vi "MTS_Main.vi"() -> ()   [LabVIEW 2010]
panel:
  out "Grid Points":dbl[][](array[numeric])
  in  "Z-Position":dbl=69.999 caption="Z" min=0.0 max=200.0 format="%1.3f um"
  in  "Y-Position":dbl=19.9997 caption="Y" min=0.0 max=200.0 format="%1.3f um"
  in  "X-Position":dbl=48.0021 caption="X" min=0.0 max=200.0 format="%1.3f um"
  in  "Move Stage":bool
  out "Detector4":bool=TRUE
  in  "Measurement Tab Control":T1(tab)
  in  "Measurement Time (s)":i32=60 min=10
  in  "Point Measurement":bool
  in  "Line Time (s)":i32=60 caption="Measurement Time (s)" min=10
  in  "Line Width":dbl=50.0 min=0.1 max=200.0 format="%1.1f um"
  in  "Line Points":u16=100
  in  "Line Scan Axis":enum32{"x-Axis", "y-Axis", "z-Axis"}(ring) caption="Axis"
  in  "Line Scan":bool
  in  "Line Scanner Divider":i32=1 caption="Scanner Divider" min=1 max=10
  in  "Grid Measurement":bool
  in  "Grid Time (s)":i32=2 caption="Time per Point (s)" min=1 max=3600
  in  "Repetitions":u16=1 min=1 max=100
  in  "Z-Axis Offset":dbl=2.0 min=0.1 max=10.0
  in  "Y-Axis Offset":dbl=2.0 min=0.1 max=10.0
  in  "X-Axis Offset":dbl=2.0 min=0.1 max=10.0
  in  "Z-Axis Points":u16=1 min=1 max=100
  in  "Y-Axis Points":u16=50 min=1 max=100
  in  "X-Axis Points":u16=50 min=1 max=100
  out "Grid Time":dbl=91.66666666666667 caption="Measurement Time (min)" format="%#_2f"
  out "Current Grid Point":i32
  in  "Axis":enum32{"x-y", "x-z", "y-z"}(ring)
  in  "Picture size 2":dbl=50.0 min=0.1 max=200.0 format="%1.1f um"
  in  "Picture size":dbl=50.0 min=0.1 max=200.0 format="%1.1f um"
  in  "Axis 2 Pixel":u16=100
  in  "Axis 1 Pixel":u16=100
  in  "Scanner Divider":i32=1 min=1 max=10
  out "Measure. time [s]":i32
  in  "Aquire Image":bool
  out "y":dbl=500.0 format="%.1f nm"
  out "x":dbl=500.0 format="%.1f nm"
  out "Detector3":bool=TRUE
  out "Counts":u32[](array[numeric])
  out "Last Image File No":i32=-1
  out "NxtAutMesPoint":i32
  out "Auto Measure Points":i32
  out "Pattern":dbl[][](array[numeric])
  out "Active pt3":path
  in  "Save Files":bool=TRUE
  out "Intensity (a.u.)":dbl=17475.78930323986 format="%.02f"
  out "Detector2":bool=TRUE
  out "Detector1":bool=TRUE
  out "Excitation":bool=TRUE
  in  "Open MSW":bool
  in  "New MSW":bool
  out "Workspace":path=path "X:/MTusers/Christoph/2011-02-01 Andi/2011-02-01.msw"
  in  "WS File Tree":string(tree)
  out "Stop Measurement":bool
  in  "Learning loop":bool=TRUE
  in  "ShowTab":T2(tab)=enum."TCSPC Histogram"
  out "Video":u8[][](graph)
  in  "Find Mols":bool
  out "Image":i32[][](graph)
  in  "Save Color Image":bool
  in  "psf width [um]":dbl=0.7
  in  "Auto Shutter Control":bool=TRUE
  out "Auto Meas Progress":i32(slide) caption="Point 8 / 15" scale=0.0..15.0
  out "AM image":T3(plugin-control)
  in  "Auto Meas":bool
  in  "Auto Measurement Time (ms)":i32=60 caption="Measurement Time (s)" min=10
  in  "Autopoint-Auto Z":bool
  out "Histogram":i32[][](graph)
  in  "CFD Settings":T4={"Sync Level"=150, "Sync ZeroX"=10, "Sync Offset"=-9000, "Chan Settings"=[{"CHx Level"=50, "CHx ZeroX"=10, "CHx Offset"=400}, {"CHx Level"=50, "CHx ZeroX"=10, "CHx Offset"=400}, {"CHx Level"=150, "CHx ZeroX"=10, "CHx Offset"=19250}, {"CHx Level"=150, "CHx ZeroX"=10, "CHx Offset"=19200}]}
  out "Trace":i32[][](graph)=[[2, 0, 0, 1, 1, 1, 0, 0, 0, 1, 0, 1, 0, 1, 2, 2, 0, 3, 0, 2, 2, 1, 3, 1, 0, 1, 1, 1, 0, 1, 3, 1, 0, 2, 0, 1, 0, 1, 1, 0, 1, 1, 3, 1, 0, 2, 0, 1, 1, 0, 0, 2, 0, 0, 1, 1, 1, 0, 0, 1, 0, 1, 0, 0, 0, 1, 2, 1, 1, 2, 0, 2, 4, 3, 1, 1, 0, 0, 1, 1, 2, 0, 1, 1, 0, 0, 0, 1, 1, 1, 1, 3, 0, 0, 1, 0, 0, 0, 2, 1, 1, 1, 2, 1, 0, 1, 1, 0, 0, 2, 1, 1, 0, 0, 1, 1, 1, 1, 0, 2, 2, 0, 1, 2, 1, 0, 3, 0, 2, 1, 3, 0, 1, 1, 0, 0, 3, 0, 0, 0, 0, 0, 0, 0, 0, 0, 0, 0, 0, 0, 0, 0, 0, 0, 0, 0, 0, 0, 0, 0, 0, 0, 0, 0, 0, 0, 0, 0, 0, 0, 0, 0, 0, 0, 0, 0, 0, 0, 0, 0, 0, 0, 0, 0, 0, 0, 0, 0, 0, 0, 0, 0, 0, 0, 0, 0, 0, 0, 0, 0], [1, 2, 2, 0, 0, 0, 1, 2, 1, 2, 1, 1, 1, 0, 0, 0, 3, 1, 0, 1, 0, 2, 0, 2, 1, 1, 0, 0, 1, 0, 1, 2, 1, 0, 0, 0, 0, 0, 1, 0, 1, 0, 2, 0, 1, 0, 0, 0, 0, 1, 1, 3, 0, 0, 0, 2, 0, 0, 2, 0, 1, 1, 0, 0, 2, 0, 2, 1, 0, 1, 1, 0, 1, 1, 0, 0, 0, 1, 0, 0, 1, 0, 0, 0, 0, 1, 0, 1, 1, 1, 1, 0, 0, 0, 1, 1, 1, 0, 1, 0, 0, 0, 1, 1, 1, 0, 0, 1, 1, 3, 1, 0, 0, 0, 0, 0, 0, 0, 1, 2, 1, 0, 0, 0, 2, 3, 3, 2, 0, 1, 1, 1, 0, 0, 4, 0, 1, 2, 0, 0, 0, 2, 0, 0, 0, 0, 0, 0, 0, 0, 0, 0, 0, 0, 0, 0, 0, 0, 0, 0, 0, 0, 0, 0, 0, 0, 0, 0, 0, 0, 0, 0, 0, 0, 0, 0, 0, 0, 0, 0, 0, 0, 0, 0, 0, 0, 0, 0, 0, 0, 0, 0, 0, 0, 0, 0, 0, 0, 0, 0], [2, 2, 0, 1, 2, 0, 1, 0, 2, 3, 1, 0, 1, 0, 1, 0, 0, 0, 0, 2, 1, 0, 0, 2, 2, 0, 0, 0, 3, 0, 0, 2, 2, 2, 0, 3, 0, 3, 1, 3, 1, 3, 1, 0, 3, 1, 3, 3, 1, 1, 1, 1, 2, 0, 1, 0, 1, 1, 1, 3, 0, 2, 3, 1, 1, 1, 0, 1, 0, 1, 2, 3, 1, 2, 1, 3, 0, 2, 0, 2, 0, 1, 0, 2, 2, 1, 1, 3, 1, 2, 1, 1, 1, 3, 0, 0, 0, 0, 1, 1, 1, 0, 1, 0, 2, 1, 1, 0, 1, 0, 1, 2, 2, 2, 2, 0, 1, 0, 0, 0, 1, 1, 2, 0, 0, 1, 5, 2, 2, 0, 2, 0, 2, 2, 2, 0, 1, 0, 6, 0, 0, 0, 0, 0, 0, 0, 0, 0, 0, 0, 0, 0, 0, 0, 0, 0, 0, 0, 0, 0, 0, 0, 0, 0, 0, 0, 0, 0, 0, 0, 0, 0, 0, 0, 0, 0, 0, 0, 0, 0, 0, 0, 0, 0, 0, 0, 0, 0, 0, 0, 0, 0, 0, 0, 0, 0, 0, 0, 0, 0], [0, 0, 1, 0, 1, 1, 0, 0, 0, 1, 1, 0, 1, 0, 0, 0, 0, 0, 2, 0, 0, 0, 0, 2, 0, 0, 0, 1, 1, 2, 1, 1, 1, 2, 1, 0, 0, 3, 0, 1, 1, 0, 0, 0, 0, 1, 0, 0, 2, 1, 0, 0, 1, 1, 1, 2, 2, 0, 1, 0, 0, 1, 0, 1, 1, 0, 0, 2, 1, 1, 2, 1, 1, 0, 0, 0, 0, 2, 1, 0, 0, 0, 0, 1, 0, 1, 0, 0, 0, 0, 1, 0, 0, 0, 0, 1, 0, 1, 1, 1, 0, 2, 3, 1, 1, 0, 1, 1, 1, 0, 1, 0, 0, 1, 1, 0, 2, 0, 0, 0, 0, 3, 0, 0, 0, 0, 0, 0, 0, 0, 1, 0, 2, 0, 0, 0, 1, 2, 2, 0, 1, 0, 0, 0, 0, 0, 0, 0, 0, 0, 0, 0, 0, 0, 0, 0, 0, 0, 0, 0, 0, 0, 0, 0, 0, 0, 0, 0, 0, 0, 0, 0, 0, 0, 0, 0, 0, 0, 0, 0, 0, 0, 0, 0, 0, 0, 0, 0, 0, 0, 0, 0, 0, 0, 0, 0, 0, 0, 0, 0]]
  out "FiFo Overrun":bool
  in  "SCANNER EMERGENCY":bool
  out "Do Measurement":T5(ring)
  in  "Settings":bool
  in  "PI E710 Port":u16(ring) items=["COM1", "COM2", "COM3", "COM4", "COM5", "COM6", "COM7", "COM8", "COM9"]
  out "MeasRunig":bool
  in  "Stop Program":bool
  out "Global Stop":bool=TRUE
  # "Workspace"
  # "Shutter:"
  # "Point Measurement Settings"
  # "Point Position"
  # "Line Scan Settings"
  # "Starting Point"
  # "Grid Measurement Settings"
  # "Starting Point"
  # "um"
  # "um"
  # "um"
  # "Image Scan Settings"
  # "Upper Left"
  # "Pixelsize"
  # "Auto Measurement Settings"
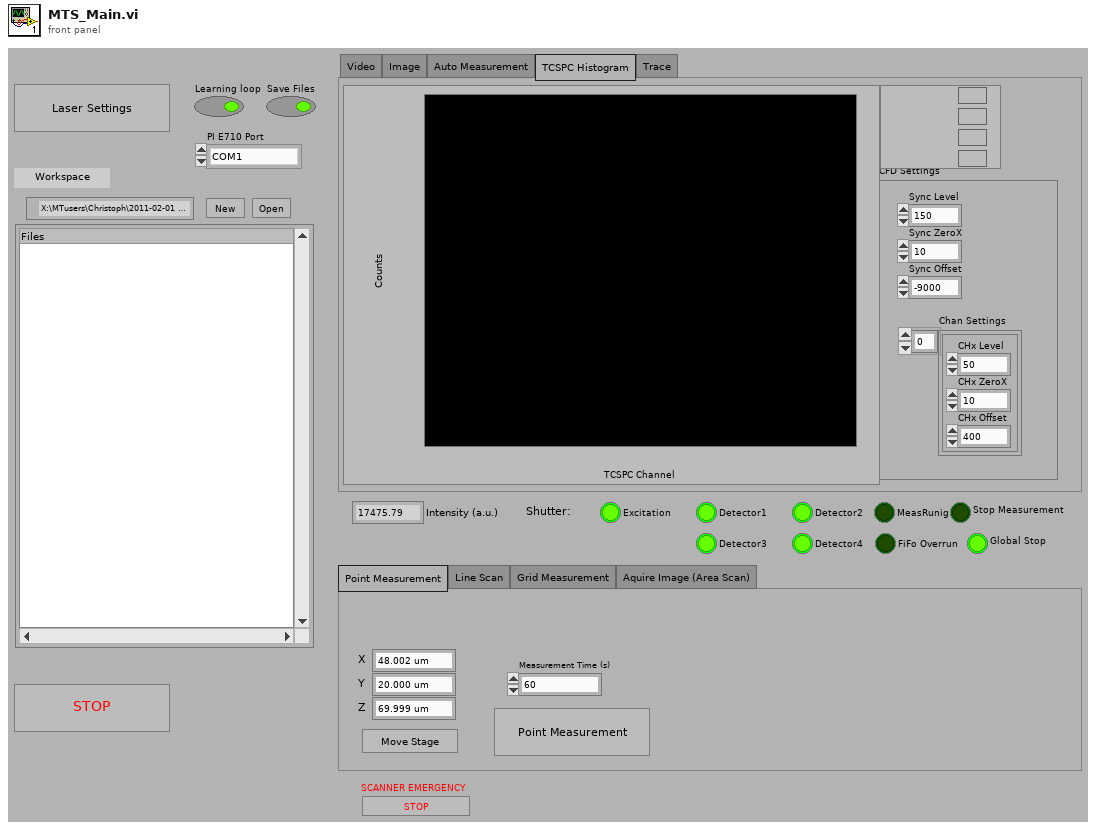
[diagram p1: front panel]
types:
  T1 = enum32{"Point Measurement", "Line Scan", "Grid Measurement", "Aquire Image (Area Scan)"}
  T2 = enum32{"Video", "Image", "Auto Measurement", "TCSPC Histogram", "Trace"}
  T3 = typedef "IMAQ Image.ctl" = refnum<image>
  T4 = cluster{"Sync Level":i32, "Sync ZeroX":i32, "Sync Offset":i32, "Chan Settings":cluster{"CHx Level":i32, "CHx ZeroX":i32, "CHx Offset":i32}[]}
  T5 = enum16{"No Measurement", "Aquire Image", "Point Measurement", "Multi Measurement", "Save Color Image", "Find Single Mol.", "Auto Measurement Control", "Auto Point", "Aquire Line Scan", "Grid Measurement"}
  T6 = cluster{"Position":cluster{"X-Position":dbl, "Y-Position":dbl, "Z-Position":dbl}, "Picture Size Axis 1":dbl, "Picture Size Axis 2":dbl, "Axis":i32, "Axis 1 Pixels":u16, "Axis 2 Pixels":u16, "Scanner Divider":i32}
  T7 = enum16{"CAN_Baud_1M", "CAN_BAUD_500K", "CAN_BAUD_250K", "CAN_BAUD_125K", "CAN_BAUD_100K", "CAN_BAUD_50K", "CAN_BAUD_20K", "CAN_BAUD_10K", "CAN_BAUD_5K", "User"}
  T8 = typedef "Image Type" = u32
  T9 = cluster{"Height":u32, "Width":u32, "Pixel Depth":u32}
  T10 = cluster{"Dev":i32, "SerNo":string, "HW_Model":string, "HW_Partno":string}[]
  T11 = enum32{"Video", "Image", "TCSPC Histogram", "Trace"}
  T12 = cluster{"ID":u32, "MSG type":enum8{"STD, NO RTR", "STD,RTR", "XTD, NO RTR", "XTD, RTR"}, "LEN":u8, "DATA":u8[]}
  T13 = enum32{"Invalid", "Standard", "Closed", "Hidden", "Minimized", "Maximized"}
  T14 = enum16{"No Measurement", "Aquire Image", "Point Measurement", "Multi Measurement", "Save Color Image"}
  T15 = enum16{"No Measurement", "Aquire Image", "Point Measurement", "Multi Measurement", "Save Color Image", "Find Single Mol.", "Auto Measurement Control", "Auto Point", "Aquire Line Scan"}
  T16 = enum16{"No Measurement", "Aquire Image", "Point Measurement", "Multi Measurement", "Save Color Image", "Find Single Mol.", "Auto Measurement Control", "Auto Point"}
  T17 = enum16{"No Measurement", "Aquire Image", "Point Measurement", "Multi Measurement", "Save Color Image", "Find Single Mol."}
  T18 = enum16{"Get (Default)", "Set Workspace", "Append File", "Change Comment"}
  T19 = enum16{"unknown", "pt3 File", "png Image", "bmp Image"}
  T20 = enum32{"Bad", "Idle", "Run top level", "Running"}
  T21 = cluster{"File No":i32, "File Path":path, "Parent File":i32, "File Type":enum16{"unknown", "pt3 File", "png Image", "bmp Image"}, "Measurement Type":enum16{"not a pt3 File", "Image File", "Point Measurement", "Auto Point", "Line Scan", "Grid Scan"}, "Upper Left":cluster{"x-Position":dbl, "y-Position":dbl, "z-Position":dbl}, "Pixels":i32[], "Picture Size":dbl[], "Scan Axis":enum32{"x-y", "x-z", "y-z"}}[]
  T22 = typedef "LVPoint32TypeDef.ctl" = cluster{"Horizontal":i32, "Vertical":i32}
  T23 = cluster{"Shift":bool, "Ctrl":bool, "Alt":bool, "Cmd":bool, "Opt":bool}
  T24 = cluster{"File No":i32, "File Path":path, "Parent File":i32, "File Type":enum16{"unknown", "pt3 File", "png Image", "bmp Image"}, "Measurement Type":enum16{"not a pt3 File", "Image File", "Point Measurement", "Auto Point", "Line Scan", "Grid Scan"}, "Upper Left":cluster{"x-Position":dbl, "y-Position":dbl, "z-Position":dbl}, "Pixels":i32[], "Picture Size":dbl[], "Scan Axis":enum32{"x-y", "x-z", "y-z"}}
  T25 = enum16{"not a pt3 File", "Image File", "Point Measurement", "Auto Point", "Line Scan", "Grid Scan"}
  T26 = cluster{"x-Position":dbl, "y-Position":dbl, "z-Position":dbl}
  T27 = cluster{"Upper Left":cluster{"x-Position":dbl, "y-Position":dbl, "z-Position":dbl}, "value":dbl, "value":dbl, "Scan Axis":enum32{"x-y", "x-z", "y-z"}, "value":i32, "value":i32, "index":i32}
  T28 = cluster{"ID":u32, "MSG type":enum8{"STD, NO RTR", "STD,RTR", "XTD, NO RTR", "XTD, RTR"}, "LEN":u8, "Data":u8[]}
  T29 = enum16{"not a pt3 File", "Image File", "Point Measurement", "Auto Point", "Line Scan"}
  T30 = enum16{"not a pt3 File", "Image File", "Point Measurement", "Auto Point"}
  T31 = cluster{"X-Position":dbl, "Y-Position":dbl, "Z-Position":dbl}
  T32 = cluster{"Dev":i32, "SerNo":string, "HW_Model":string, "HW_Partno":string}
  T33 = cluster{"Comment":string, "Binning":i32, "Offset":i32, "AcquisitionTime (ms)":i32, "HardwareSerial":i32, "SyncDivider":i32, "Resolution (ps)":dbl, "InpRate0":i32, "InpRate1":i32, "CFD Settings":cluster{"Sync Level":i32, "Sync ZeroX":i32, "Sync Offset":i32, "Chan Settings":cluster{"CHx Level":i32, "CHx ZeroX":i32, "CHx Offset":i32}[]}, "ModuleInfo":cluster{"modelcode":i32, "versioncode":i32}[], "BaseResolution (ps)":dbl, "RefClockSource":i32, "ChanInfo":cluster{"CHx Level":i32, "CHx ZeroX":i32, "CHx Offset":i32, "CHx modidx":i32}[], "SyncRate":i32, "InputsEnabled":i64}
  T34 = cluster{"Dimensions":i32, "Time Per Pixel [ms]":dbl, "Acceleration":i32, "Pattern":i32, "X0":sgl, "Y0":sgl, "PixX":i32, "PixY":i32, "PixResol":sgl, "TStartTo":sgl, "TStoptTo":sgl, "TStartFro":sgl, "TStopFro":sgl}
  T35 = cluster{"InpRateFilePos":i64, "StopAfterFilePos":i64}
  T36 = cluster{"Picture Size":dbl[], "Pixels":i32[], "Upper Left":cluster{"x-Position":dbl, "y-Position":dbl, "z-Position":dbl}}
  T37 = cluster{"Ident":string, "Format Version":string, "Creator Name":string, "Creator Version":string, "File Time":string, "Comment":string, "Binning":i32, "Offset":i32, "AcquisitionTime (ms)":i32, "HardwareSerial":i32, "SyncDivider":i32, "Resolution (ps)":dbl, "InpRate0":i32, "InpRate1":i32, "CFD Settings":cluster{"Sync Level":i32, "Sync ZeroX":i32, "Sync Offset":i32, "Chan Settings":cluster{"CHx Level":i32, "CHx ZeroX":i32, "CHx Offset":i32}[]}}
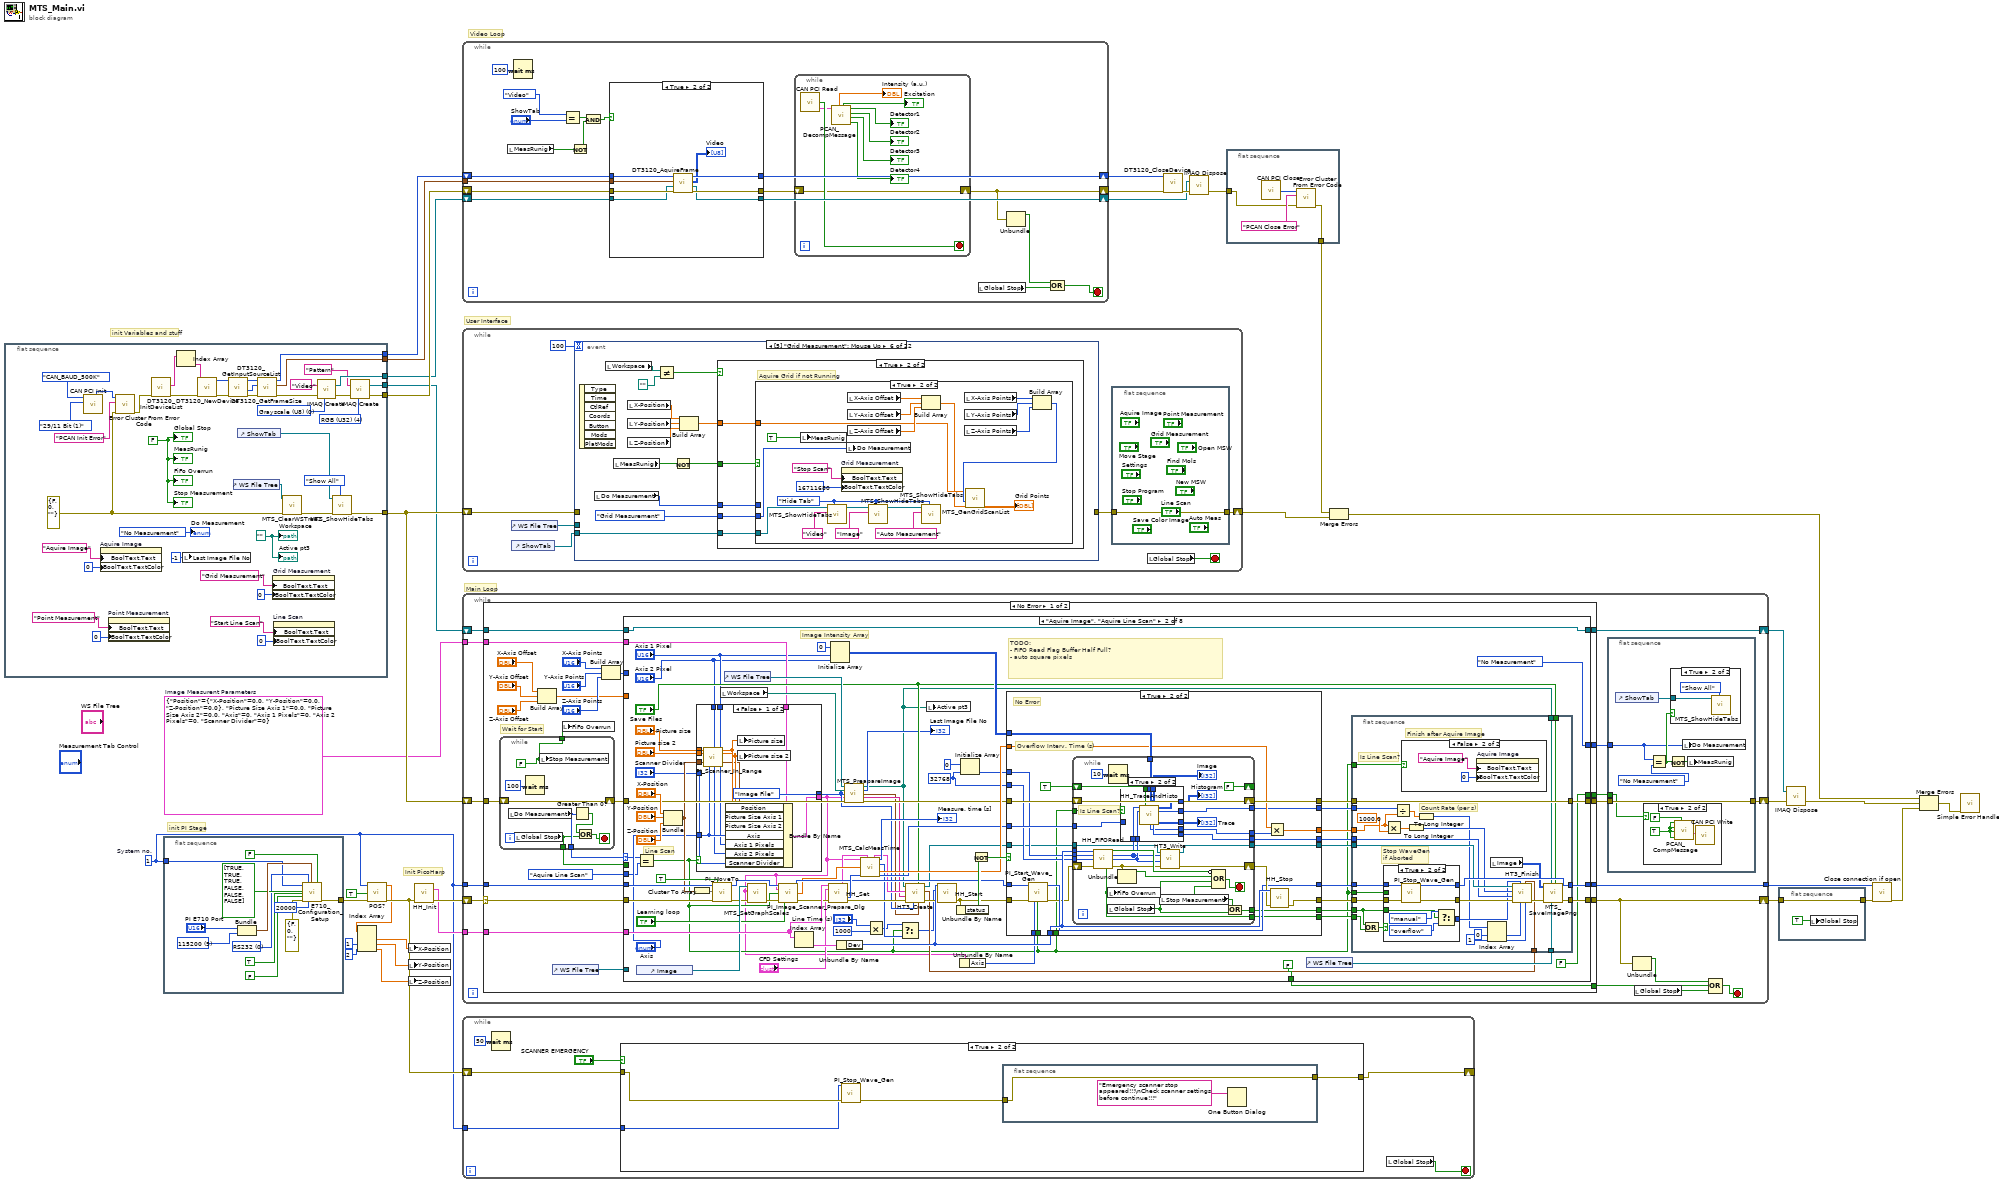
[diagram p0: block diagram]
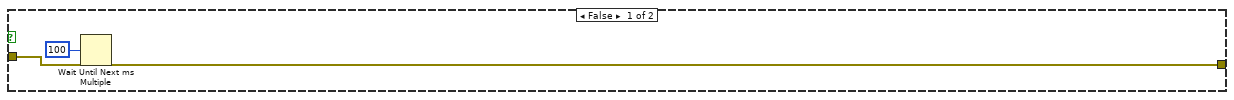
[diagram p3: hidden frame]
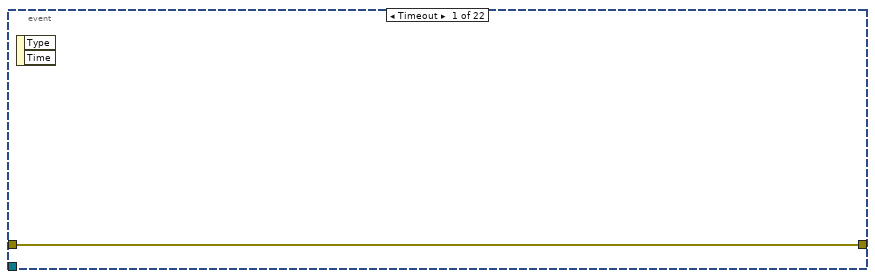
[diagram p4: hidden frame]
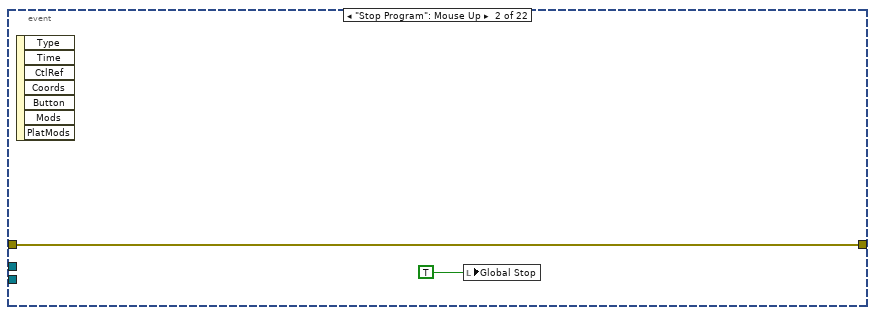
[diagram p5: hidden frame]
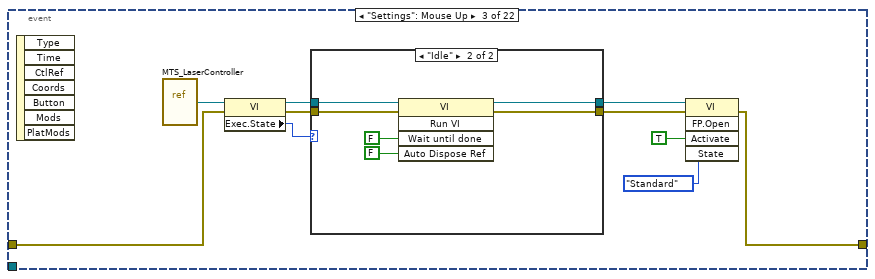
[diagram p6: hidden frame]
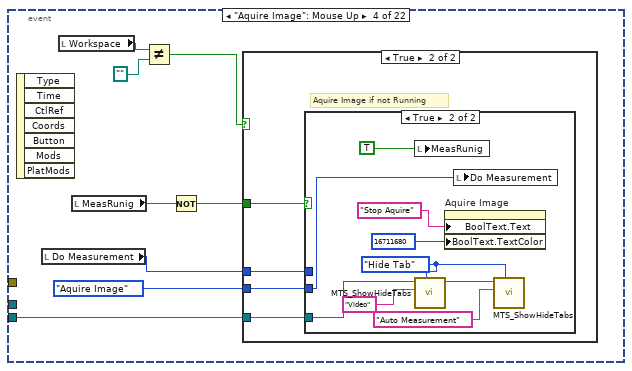
[diagram p8: hidden frame]
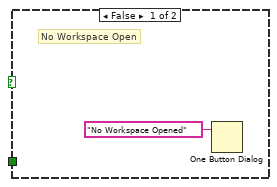
[diagram p9: hidden frame]
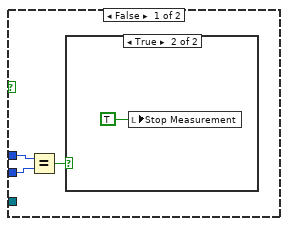
[diagram p10: hidden frame]
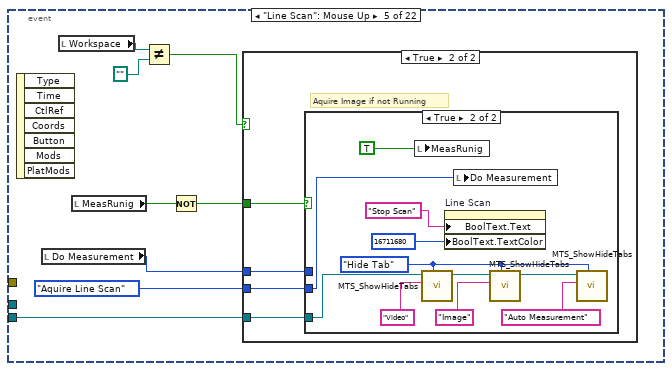
[diagram p12: hidden frame]
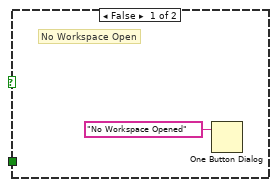
[diagram p13: hidden frame]
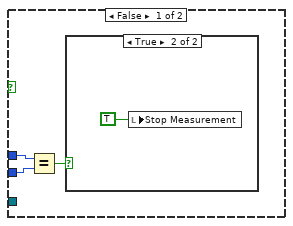
[diagram p14: hidden frame]
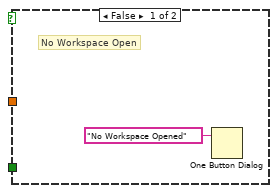
[diagram p16: hidden frame]
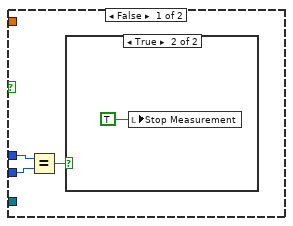
[diagram p17: hidden frame]
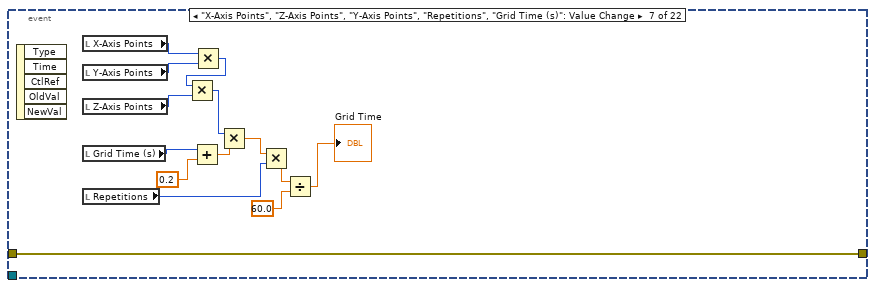
[diagram p19: hidden frame]
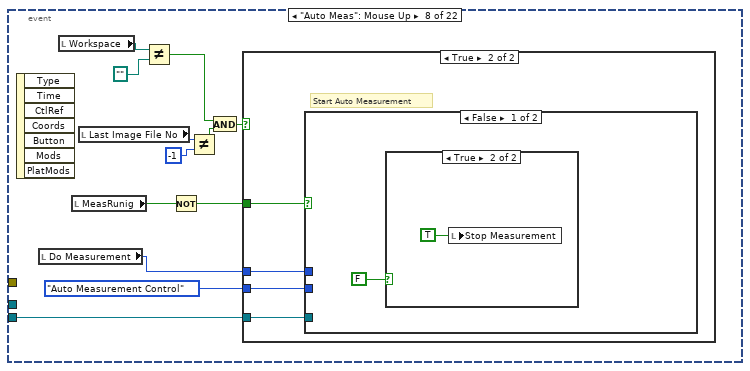
[diagram p20: hidden frame]
diagram:
  w1 = T6 {"Position"={"X-Position"=0.0, "Y-Position"=0.0, "Z-Position"=0.0}, "Picture Size Axis 1"=0.0, "Picture Size Axis 2"=0.0, "Axis"=0, "Axis 1 Pixels"=0, "Axis 2 Pixels"=0, "Scanner Divider"=0}  # Image Measurent Parameters
  w8 = 1  # System no.
  # "Video Loop"
  # "Init PicoHarp"
  # "init Variables and stuff"
  # "User Interface"
  # "init PI Stage"
  # "Main Loop"
  n1 = flat-sequence {
    tunnel: [w61] -> w32
    tunnel: [w51] -> w27
    tunnel: [w68] -> w25
    tunnel: [w65] -> w21
    tunnel: [w50] -> w20
    tunnel: [w47] -> w12
    frame #0 {
      w48 = T8 4 items=["Grayscale (U8)", "Grayscale (I16)", "Grayscale (SGL)", "Complex (CSG)", "RGB (U32)", "HSL (U32)", "RGB (U64)", "Grayscale (U16)"] ("Image Type")
      w66 = T8 0 items=["Grayscale (U8)", "Grayscale (I16)", "Grayscale (SGL)", "Complex (CSG)", "RGB (U32)", "HSL (U32)", "RGB (U64)", "Grayscale (U16)"] ("Image Type")
      w41 = path ""
      w55 = errorcluster {"status"=FALSE, "code"=0, "source"=""} ("error in")
      w77 = FALSE ("Global Stop")
      n2 = call "CAN PCI Init.vi"("CAN Msg Type"=enum16{"11 Bit (0)", "29/11 Bit (1)"}."29/11 Bit (1)", "BTR0BTR1"=T7."CAN_BAUD_500K") -> ("Error Number"=w56:u32)  [unwired: 7 in, 2 out]
      n3 = property on="Aquire Image" class="Bool"("BoolText.Text"="Aquire Image" ("Caption.Text"), "BoolText.TextColor"=u32 0 ("Boolean Text.Colors:FG Color")) -> ()  [unwired: 2 in, 2 out]
      n4 = property on="Point Measurement" class="Bool"("BoolText.Text"="Point Measurement" ("Caption.Text"), "BoolText.TextColor"=u32 0 ("Boolean Text.Colors:FG Color")) -> ()  [unwired: 2 in, 2 out]
      n5 = call <vilib>:"Error Cluster From Error Code.vi"("error in (no error)"=w55, "error message (\"\")"="PCAN Init Error" ("error message (\"\")"), "error code (0)"=w56) -> ("error out"=w54:errorcluster)  [unwired: 6 in]
      n6 = call "DT3120_InitDeviceList.vi"("error in (no error)"=w54) -> ("error out"=w75:errorcluster, "Alias List"=w76:string[])  [unwired: 9 out]
      n7 = Index Array(array=w76) -> (element=w74:string)  [unwired: 1 in]
      n8 = local write "Last Image File No"(-1 ("Last Image File No")) -> ()
      n9 = call "DT3120_NewDevice.vi"("error in (no error)"=w75, "Alias"=w74) -> ("error out"=w70:errorcluster, "DevId"=w69:i32)  [unwired: 8 out]
      n10 = call "DT3120_GetInputSourceList.vi"("error in (no error)"=w70, "DevId"=w69) -> ("error out"=w73:errorcluster, "Active Source"=w72:u16, "DevId (dup)"=w71:i32)  [unwired: 7 out]
      n11 = control-ref of="WS File Tree"() -> (w63:refnum<vi>)
      n12 = control-ref of="ShowTab"() -> (w60:refnum<vi>)
      n13 = call "DT3120_GetFrameSize.vi"("error in (no error)"=w73, "Source"=w72, "DevId"=w71) -> ("error out"=w67:errorcluster, "Frame Size"=w65:T9, "DevId (dup)"=w68:i32)  [unwired: 6 in]
      n14 = property on="Grid Measurement" class="Bool"("BoolText.Text"="Grid Measurement" ("Caption.Text"), "BoolText.TextColor"=u32 0 ("Boolean Text.Colors:FG Color")) -> ()  [unwired: 2 in, 2 out]
      n15 = property on="Line Scan" class="Bool"("BoolText.Text"="Start Line Scan" ("Caption.Text"), "BoolText.TextColor"=u32 0 ("Boolean Text.Colors:FG Color")) -> ()  [unwired: 2 in, 2 out]
      n16 = call "MTS_ClearWSTree2.vi"("error in"=w55, "Tree Refnum"=w63) -> ("error out"=w62:errorcluster)  [unwired: 8 in, 1 out]
      n17 = call "IMAQ Create"("Image Name"="Video", "Image Type"=w66, "error in (no error)"=w67) -> ("New Image"=w50:T3, "error out"=w52:errorcluster)  [unwired: 2 in]
      n18 = call "MTS_ShowHideTabs.vi"("Action"=enum16{"Show All", "Hide Tab", "Show Tab"}."Show All", "error in (no error)"=w62, "ShowTab"=w60) -> ("error out"=w61:errorcluster)  [unwired: 7 in, 1 out]
      n19 = call "IMAQ Create"("Image Name"="Pattern", "Image Type"=w48, "error in (no error)"=w52) -> ("New Image"=w47:T3, "error out"=w51:errorcluster)  [unwired: 2 in]
      "Global Stop" <- w77
      "MeasRunig" <- w77
      "Do Measurement" <- T5."No Measurement" ("Do Measurement")
      "FiFo Overrun" <- w77
      "Stop Measurement" <- w77
      "Workspace" <- w41
      "Active pt3" <- w41
    }
  }
  n20 = flat-sequence {
    tunnel: [w81] -> w11
    tunnel: w8 -> [w80]
    frame #0 {
      w88 = u16 5 items=["9600", "14400", "19200", "38400", "57600", "115200"] ("Baudrate")
      w83 = u16 0 items=["RS232", "GPIB"] ("Interface")
      n21 = Bundle("PI E710 Port"="PI E710 Port", "Baudrate"=w88) -> (w89:cluster{"PI E710 Port":u16, "Baudrate":u16})  [unwired: 1 out]
      n22 = call <userlib>:"E710_Configuration_Setup.vi"("System no."=w80, "Are stages connected?"=bool[] [TRUE, TRUE, TRUE, FALSE, FALSE, FALSE], "Change servo \nstatus to ON?"=TRUE ("Change servo \nstatus to ON?"), "Perform autozero?"=FALSE ("All axes?"), "error in"=errorcluster {"status"=FALSE, "code"=0, "source"=""}, "Interface"=w83, "Timeout"=u32 20000, "RS232 settings"=w89, "Move to middle?"=FALSE) -> ("error out"=w81:errorcluster)  [unwired: 3 in, 7 out]
    }
  }
  n23 = call <userlib>:"POS?.vi"("System no."=w8, "All axes?"=TRUE, "error in"=w11) -> ("Position"=w7:dbl[], "error out"=w10:errorcluster)  [unwired: 2 in, 13 out]
  n24 = Index Array(array=w7, index #2=1 ("index"), index #3=2 ("index")) -> (element #1=w3:dbl, element #2=w2:dbl, element #3=w4:dbl)  [unwired: 1 in]
  n25 = local write "X-Position"(w3) -> ()
  n26 = local write "Y-Position"(w2) -> ()
  n27 = local write "Z-Position"(w4) -> ()
  n28 = call "HH_Init.vi"("error in (no error)"=w10) -> ("Device List"=w30:T10, "error out"=w31:errorcluster)  [unwired: 12 in, 1 out]
  n29 = while {
    shift-right: [w90] -> w26
    shift-left: w27 -> [w104]
    shift-right: [w97] -> w24
    shift-left: w25 -> [w98]
    tunnel: w21 -> [w99]
    shift-right: [w96] -> w18
    shift-left: w20 -> [w100]
    stop <- w103 stop-if-true
    n30 = local read "MeasRunig"() -> (w95:bool)
    n31 = Wait (ms)(milliseconds to wait=u32 100) -> ()  [unwired: 1 out]
    n32 = Equal?(x=T11."Video" ("ShowTab"), y="ShowTab") -> (x = y?=w94:bool)
    n33 = Not(x=w95) -> (.not. x?=w92:bool)
    n34 = And(x=w94, y=w92) -> (x .and. y?=w93:bool)
    n35 = case shown="True" w93 {
      tunnel: w104 -> [w119 w127]
      tunnel: [w119 w126] -> w91
      tunnel: w100 -> [w117 w125]
      tunnel: w99 -> [_ w124]
      tunnel: w98 -> [w118 w123]
      tunnel: [w118 w122] -> w97
      tunnel: [w117 w121] -> w96
      frame False {
      }
      frame True {
        n36 = call "DT3120_AquireFrame.vi"("error in (no error)"=w127, "Image"=w125, "Frame Size"=w124, "DevId"=w123) -> ("error out"=w126:errorcluster, "Image Out"=w121:T3, "Frame"=→"Video":u8[][], "DevId (dup)"=w122:i32)  [unwired: 4 in]
      }
    }
    n37 = while {
      shift-right: [w114] -> w90
      shift-left: w91 -> [w114]
      stop <- w116 stop-if-true
      n38 = call "CAN PCI Read.vi"() -> ("RcvQueueEmpty"=w116:bool, "CAN_Message out"=w115:T12)  [unwired: 1 in, 1 out]
      n39 = call "PCAN_DecompMessage.vi"("CAN_Message out"=w115) -> ("Detector4 Shutter Open?"=→"Detector4":bool, "Detector3 Shutter Open?"=→"Detector3":bool, "Detector2 Shutter Open?"=→"Detector2":bool, "Detector1 Shutter Open?"=→"Detector1":bool, "Excitation Shutter Open?"=→"Excitation":bool, "Intensity (a.u.)"=→"Intensity (a.u.)":dbl)  [unwired: 3 in, 2 out]
    }
    n40 = local read "Global Stop"() -> (w102:bool)
    n41 = Unbundle(w90) -> ("status"=w101:bool)  [unwired: 2 out]
    n42 = Compound Arithmetic op=OR(w101, w102) -> (w103:bool)
  }
  n43 = while {
    shift-right: [w132] -> w23
    shift-left: w32 -> [w133]
    stop <- w130 stop-if-true
    n44 = control-ref of="WS File Tree"() -> (w129:refnum<vi>)
    n45 = control-ref of="ShowTab"() -> (w128:refnum<vi>)
    n46 = event shown="[5] \"Grid Measurement\": Mouse Up" {
      selector: _ -> [_ _ _ _ _ _ _ _ _ _ _ _ _ _ _ _ _ _ _ _ _ _]
      dyn-events: _ -> [_ _ _ _ _ _ _ _ _ _ _ _ _ _ _ _ _ _ _ _ _ _]
      timeout: 100 -> [_ _ _ _ _ _ _ _ _ _ _ _ _ _ _ _ _ _ _ _ _ _]
      tunnel: w133 -> [w136 w138 w147 _ _ _ w267 _ _ _ _ _ w354 w390 _ w442 _ _ _ _ _ _]
      tunnel: [w136 w138 w139 _ _ _ w267 _ _ _ _ _ w352 w387 _ w441 _ _ _ _ _ _] -> w131
      tunnel: w129 -> [_ _ _ _ _ _ _ _ _ _ _ _ w356 w391 _ _ _ _ _ _ _ _]
      tunnel: w128 -> [_ _ _ w157 w184 w216 _ w274 w293 w301 w309 w337 _ _ _ _ _ _ _ _ _ _]
      event Timeout {
        n47 = event-data() -> ()  [unwired: 1 in, 2 out]
      }
      event "Stop Program": Mouse Up {
        n48 = event-data() -> ()  [unwired: 1 in, 7 out]
        n49 = local write "Global Stop"(TRUE ("Global Stop")) -> ()
      }
      event "Settings": Mouse Up {
        n50 = event-data() -> ()  [unwired: 1 in, 7 out]
        n51 = vi-ref "MTS_LaserController.vi"() -> (w148:refnum<vi>)
        n52 = property class="VI"(reference=w148, error in=w147) -> (reference out=w145:refnum<vi>, error out=w146:errorcluster, "Exec.State"=w144:T20)
        n53 = case shown="\"Idle\"" w144 {
          tunnel: w146 -> [w150 w156]
          tunnel: w145 -> [w149 w155]
          tunnel: [w150 w152] -> w143
          tunnel: [w149 w151] -> w142
          frame "Bad", Default {
          }
          frame "Idle" {
            n54 = invoke class="VI" method="Run VI"(reference=w155, error in=w156, "Wait until done"=FALSE ("Wait Until Done"), "Auto Dispose Ref"=FALSE ("Auto Dispose Reference")) -> (reference out=w151:refnum<vi>, error out=w152:errorcluster)  [unwired: 1 in, 3 out]
          }
        }
        n55 = invoke class="VI" method="FP.Open"(reference=w142, error in=w143, "Activate"=TRUE ("Activate?"), "State"=T13."Standard") -> (error out=w139:errorcluster)  [unwired: 1 in, 4 out]
      }
      event "Aquire Image": Mouse Up {
        n56 = event-data() -> ()  [unwired: 1 in, 7 out]
        n57 = local read "Do Measurement"() -> (w161:T5)
        n58 = local read "Workspace"() -> (w160:path)
        n59 = local read "MeasRunig"() -> (w164:bool)
        n60 = Not Equal?(x=w160, y=path "") -> (x != y?=w158:bool)
        n61 = Not(x=w164) -> (.not. x?=w163:bool)
        n62 = case shown="True" w158 {
          tunnel: w163 -> [_ w169]
          tunnel: T14."Aquire Image" ("Do Measurement") -> [_ w168]
          tunnel: w161 -> [_ w167]
          tunnel: w157 -> [_ w166]
          frame False {
            # "No Workspace Open"
            n63 = One Button Dialog(message="No Workspace Opened") -> ()  [unwired: 1 in, 1 out]
          }
          frame True {
            # "Aquire Image if not Running"
            n64 = case shown="True" w169 {
              tunnel: w168 -> [w171 w180]
              tunnel: w167 -> [w172 _]
              tunnel: w166 -> [_ w177]
              frame False {
                n65 = Equal?(x=w172, y=w171) -> (x = y?=w170:bool)
                n66 = case shown="True" w170 {
                  frame False {
                  }
                  frame True {
                    n67 = local write "Stop Measurement"(TRUE ("Stop Measurement")) -> ()
                  }
                }
              }
              frame True {
                w175 = enum16{"Show All", "Hide Tab", "Show Tab"}."Hide Tab" ("Action")
                n68 = local write "MeasRunig"(TRUE ("Measurement Running")) -> ()
                n69 = call "MTS_ShowHideTabs.vi"("Action"=w175, "Tab Caption"="Video", "ShowTab"=w177) -> ("ShowTab (dup)"=w176:refnum<vi>)  [unwired: 7 in, 1 out]
                n70 = property on="Aquire Image" class="Bool"("BoolText.Text"="Stop Aquire" ("Caption.Text"), "BoolText.TextColor"=u32 16711680 ("Boolean Text.Colors:FG Color")) -> ()  [unwired: 2 in, 2 out]
                n71 = local write "Do Measurement"(w180) -> ()
                n72 = call "MTS_ShowHideTabs.vi"("Action"=w175, "Tab Caption"="Auto Measurement", "ShowTab"=w176) -> ()  [unwired: 7 in, 2 out]
              }
            }
          }
        }
      }
      event "Line Scan": Mouse Up {
        n73 = event-data() -> ()  [unwired: 1 in, 7 out]
        n74 = local read "Do Measurement"() -> (w188:T5)
        n75 = local read "Workspace"() -> (w187:path)
        n76 = local read "MeasRunig"() -> (w190:bool)
        n77 = Not Equal?(x=w187, y=path "") -> (x != y?=w185:bool)
        n78 = Not(x=w190) -> (.not. x?=w189:bool)
        n79 = case shown="True" w185 {
          tunnel: w189 -> [_ w195]
          tunnel: T15."Aquire Line Scan" ("Do Measurement") -> [_ w194]
          tunnel: w188 -> [_ w193]
          tunnel: w184 -> [_ w192]
          frame False {
            # "No Workspace Open"
            n80 = One Button Dialog(message="No Workspace Opened") -> ()  [unwired: 1 in, 1 out]
          }
          frame True {
            # "Aquire Image if not Running"
            n81 = case shown="True" w195 {
              tunnel: w194 -> [w197 w208]
              tunnel: w193 -> [w198 _]
              tunnel: w192 -> [_ w205]
              frame False {
                n82 = Equal?(x=w198, y=w197) -> (x = y?=w196:bool)
                n83 = case shown="True" w196 {
                  frame False {
                  }
                  frame True {
                    n84 = local write "Stop Measurement"(TRUE ("Stop Measurement")) -> ()
                  }
                }
              }
              frame True {
                w200 = enum16{"Show All", "Hide Tab", "Show Tab"}."Hide Tab" ("Action")
                n85 = local write "MeasRunig"(TRUE ("Measurement Running")) -> ()
                n86 = call "MTS_ShowHideTabs.vi"("Action"=w200, "Tab Caption"="Video", "ShowTab"=w205) -> ("ShowTab (dup)"=w203:refnum<vi>)  [unwired: 7 in, 1 out]
                n87 = property on="Line Scan" class="Bool"("BoolText.Text"="Stop Scan" ("Caption.Text"), "BoolText.TextColor"=u32 16711680 ("Boolean Text.Colors:FG Color")) -> ()  [unwired: 2 in, 2 out]
                n88 = local write "Do Measurement"(w208) -> ()
                n89 = call "MTS_ShowHideTabs.vi"("Action"=w200, "Tab Caption"="Image", "ShowTab"=w203) -> ("ShowTab (dup)"=w201:refnum<vi>)  [unwired: 7 in, 1 out]
                n90 = call "MTS_ShowHideTabs.vi"("Action"=w200, "Tab Caption"="Auto Measurement", "ShowTab"=w201) -> ()  [unwired: 7 in, 2 out]
              }
            }
          }
        }
      }
      event "Grid Measurement": Mouse Up {
        n91 = event-data() -> ()  [unwired: 1 in, 7 out]
        n92 = local read "Do Measurement"() -> (w220:T5)
        n93 = local read "Workspace"() -> (w219:path)
        n94 = local read "MeasRunig"() -> (w222:bool)
        n95 = local read "X-Position"() -> (w212:dbl)
        n96 = local read "Y-Position"() -> (w213:dbl)
        n97 = local read "Z-Position"() -> (w214:dbl)
        n98 = Not Equal?(x=w219, y=path "") -> (x != y?=w217:bool)
        n99 = Not(x=w222) -> (.not. x?=w221:bool)
        n100 = Build Array(w212, w213, w214) -> (w211:dbl[])
        n101 = case shown="True" w217 {
          tunnel: w221 -> [_ w228]
          tunnel: T5."Grid Measurement" ("Do Measurement") -> [_ w227]
          tunnel: w220 -> [_ w226]
          tunnel: w216 -> [_ w225]
          tunnel: w211 -> [_ w224]
          frame False {
            # "No Workspace Open"
            n102 = One Button Dialog(message="No Workspace Opened") -> ()  [unwired: 1 in, 1 out]
          }
          frame True {
            # "Aquire Grid if not Running"
            n103 = case shown="True" w228 {
              tunnel: w227 -> [w230 w251]
              tunnel: w226 -> [w231 _]
              tunnel: w225 -> [_ w248]
              tunnel: w224 -> [_ w234]
              frame False {
                n104 = Equal?(x=w231, y=w230) -> (x = y?=w229:bool)
                n105 = case shown="True" w229 {
                  frame False {
                  }
                  frame True {
                    n106 = local write "Stop Measurement"(TRUE ("Stop Measurement")) -> ()
                  }
                }
              }
              frame True {
                w243 = enum16{"Show All", "Hide Tab", "Show Tab"}."Hide Tab" ("Action")
                n107 = local write "MeasRunig"(TRUE ("Measurement Running")) -> ()
                n108 = call "MTS_ShowHideTabs.vi"("Action"=w243, "Tab Caption"="Video", "ShowTab"=w248) -> ("ShowTab (dup)"=w246:refnum<vi>)  [unwired: 7 in, 1 out]
                n109 = property on="Grid Measurement" class="Bool"("BoolText.Text"="Stop Scan" ("Caption.Text"), "BoolText.TextColor"=u32 16711680 ("Boolean Text.Colors:FG Color")) -> ()  [unwired: 2 in, 2 out]
                n110 = local write "Do Measurement"(w251) -> ()
                n111 = local read "X-Axis Offset"() -> (w242:dbl)
                n112 = local read "Y-Axis Offset"() -> (w241:dbl)
                n113 = local read "Z-Axis Offset"() -> (w240:dbl)
                n114 = call "MTS_ShowHideTabs.vi"("Action"=w243, "Tab Caption"="Image", "ShowTab"=w246) -> ("ShowTab (dup)"=w244:refnum<vi>)  [unwired: 7 in, 1 out]
                n115 = Build Array(w242, w241, w240) -> (w233:dbl[])
                n116 = call "MTS_ShowHideTabs.vi"("Action"=w243, "Tab Caption"="Auto Measurement", "ShowTab"=w244) -> ()  [unwired: 7 in, 2 out]
                n117 = local read "X-Axis Points"() -> (w239:u16)
                n118 = local read "Y-Axis Points"() -> (w238:u16)
                n119 = local read "Z-Axis Points"() -> (w237:u16)
                n120 = Build Array(w239, w238, w237) -> (w235:u16[])
                n121 = call "MTS_GenGridScanList.vi"("Offsets"=w233, "Points"=w235, "Starting"=w234) -> ("Grid Points"=→"Grid Points":dbl[][])  [unwired: 8 in]
              }
            }
          }
        }
      }
      event "X-Axis Points", "Z-Axis Points", "Y-Axis Points", "Repetitions", "Grid Time (s)": Value Change {
        n122 = event-data() -> ()  [unwired: 1 in, 5 out]
        n123 = local read "X-Axis Points"() -> (w266:u16)
        n124 = local read "Y-Axis Points"() -> (w265:u16)
        n125 = local read "Z-Axis Points"() -> (w264:u16)
        n126 = local read "Grid Time (s)"() -> (w260:i32)
        n127 = local read "Repetitions"() -> (w257:u16)
        n128 = Add(x=w260, y=0.2) -> (x+y=w259:dbl)
        n129 = Multiply(x=w266, y=w265) -> (x*y=w263:u16)
        n130 = Multiply(x=w263, y=w264) -> (x*y=w262:u16)
        n131 = Multiply(x=w262, y=w259) -> (x*y=w258:dbl)
        n132 = Multiply(x=w258, y=w257) -> (x*y=w256:dbl)
        n133 = Divide(x=w256, y=60.0) -> (x/y=→"Grid Time":dbl)
      }
      event "Auto Meas": Mouse Up {
        n134 = event-data() -> ()  [unwired: 1 in, 7 out]
        n135 = local read "Do Measurement"() -> (w277:T5)
        n136 = local read "Workspace"() -> (w276:path)
        n137 = local read "MeasRunig"() -> (w279:bool)
        n138 = local read "Last Image File No"() -> (w272:i32)
        n139 = Not Equal?(x=w276, y=path "") -> (x != y?=w270:bool)
        n140 = Not(x=w279) -> (.not. x?=w278:bool)
        n141 = Not Equal?(x=w272, y=-1) -> (x != y?=w269:bool)
        n142 = And(x=w270, y=w269) -> (x .and. y?=w268:bool)
        n143 = case shown="True" w268 {
          tunnel: w278 -> [_ w284]
          tunnel: T16."Auto Measurement Control" ("Do Measurement") -> [_ w283]
          tunnel: w277 -> [_ w282]
          tunnel: w274 -> [_ w281]
          frame False {
            # "No Workspace Open"
            n144 = One Button Dialog(message="No Workspace Opened or No Image Acquired") -> ()  [unwired: 1 in, 1 out]
          }
          frame True {
            # "Start Auto Measurement"
            n145 = case shown="False" w284 {
              tunnel: w283 -> [_ w291]
              tunnel: w282 -> [_ _]
              tunnel: w281 -> [_ w288]
              frame False {
                n146 = case shown="True" FALSE {
                  frame False {
                  }
                  frame True {
                    n147 = local write "Stop Measurement"(TRUE ("Stop Measurement")) -> ()
                  }
                }
              }
              frame True {
                n148 = local write "MeasRunig"(TRUE ("Measurement Running")) -> ()
                n149 = local write "Do Measurement"(w291) -> ()
                n150 = call "MTS_ShowHideTabs.vi"("Action"=enum16{"Show All", "Hide Tab", "Show Tab"}."Hide Tab", "Tab Caption"="Video", "ShowTab"=w288) -> ()  [unwired: 7 in, 2 out]
                n151 = local write "NxtAutMesPoint"(-1 ("Next Auto Measure Point")) -> ()
              }
            }
          }
        }
      }
      event "Save Color Image": Mouse Up {
        n152 = event-data() -> ()  [unwired: 1 in, 7 out]
        n153 = local read "Active pt3"() -> (w296:path)
        n154 = Not Equal?(x=w296, y=path "") -> (x != y?=w294:bool)
        n155 = case shown="True" w294 {
          tunnel: T17."Save Color Image" ("Do Measurement") -> [_ w300]
          tunnel: w293 -> [_ _]
          frame False {
            # "No Workspace Open"
            n156 = One Button Dialog(message="No pt3 File opened") -> ()  [unwired: 1 in, 1 out]
          }
          frame True {
            # "Aquire Image if not Running"
            n157 = local write "MeasRunig"(TRUE ("Measurement Running")) -> ()
            n158 = local write "Do Measurement"(w300) -> ()
          }
        }
      }
      event "Find Mols": Mouse Up {
        n159 = event-data() -> ()  [unwired: 1 in, 7 out]
        n160 = local read "Active pt3"() -> (w304:path)
        n161 = Not Equal?(x=w304, y=path "") -> (x != y?=w302:bool)
        n162 = case shown="True" w302 {
          tunnel: T17."Find Single Mol." ("Do Measurement") -> [_ w308]
          tunnel: w301 -> [_ _]
          frame False {
            # "No Workspace Open"
            n163 = One Button Dialog(message="No pt3 File opened") -> ()  [unwired: 1 in, 1 out]
          }
          frame True {
            # "Aquire Image if not Running"
            n164 = local write "MeasRunig"(TRUE ("Measurement Running")) -> ()
            n165 = local write "Do Measurement"(w308) -> ()
          }
        }
      }
      event "Point Measurement": Mouse Up {
        n166 = event-data() -> ()  [unwired: 1 in, 7 out]
        n167 = local read "Do Measurement"() -> (w313:T5)
        n168 = local read "Workspace"() -> (w312:path)
        n169 = local read "MeasRunig"() -> (w316:bool)
        n170 = Not Equal?(x=w312, y=path "") -> (x != y?=w310:bool)
        n171 = Not(x=w316) -> (.not. x?=w315:bool)
        n172 = case shown="True" w310 {
          tunnel: w315 -> [_ w321]
          tunnel: T14."Point Measurement" ("Do Measurement") -> [_ w320]
          tunnel: w313 -> [_ w319]
          tunnel: w309 -> [_ w318]
          frame False {
            # "No Workspace Open"
            n173 = One Button Dialog(message="No Workspace Opened") -> ()  [unwired: 1 in, 1 out]
          }
          frame True {
            # "Aquire Image if not Running"
            n174 = case shown="True" w321 {
              tunnel: w320 -> [w323 w334]
              tunnel: w319 -> [w324 _]
              tunnel: w318 -> [_ w326]
              frame False {
                n175 = Equal?(x=w324, y=w323) -> (x = y?=w322:bool)
                n176 = case shown="True" w322 {
                  frame False {
                  }
                  frame True {
                    n177 = local write "Stop Measurement"(TRUE ("Stop Measurement")) -> ()
                  }
                }
              }
              frame True {
                w327 = enum16{"Show All", "Hide Tab", "Show Tab"}."Hide Tab" ("Action")
                n178 = local write "MeasRunig"(TRUE ("Measurement Running")) -> ()
                n179 = call "MTS_ShowHideTabs.vi"("Action"=w327, "Tab Caption"="Video", "ShowTab"=w326) -> ("ShowTab (dup)"=w330:refnum<vi>)  [unwired: 7 in, 1 out]
                n180 = property on="Point Measurement" class="Bool"("BoolText.Text"="Stop Aquire" ("Caption.Text"), "BoolText.TextColor"=u32 16711680 ("Boolean Text.Colors:FG Color")) -> ()  [unwired: 2 in, 2 out]
                n181 = local write "Do Measurement"(w334) -> ()
                n182 = call "MTS_ShowHideTabs.vi"("Action"=w327, "Tab Caption"="Image", "ShowTab"=w330) -> ("ShowTab (dup)"=w328:refnum<vi>)  [unwired: 7 in, 1 out]
                n183 = call "MTS_ShowHideTabs.vi"("Action"=w327, "Tab Caption"="Auto Measurement", "ShowTab"=w328) -> ()  [unwired: 7 in, 2 out]
              }
            }
          }
        }
      }
      event "Move Stage": Mouse Up {
        n184 = event-data() -> ()  [unwired: 1 in, 7 out]
        n185 = local read "Do Measurement"() -> (w341:T5)
        n186 = local read "Workspace"() -> (w340:path)
        n187 = local read "MeasRunig"() -> (w344:bool)
        n188 = Not Equal?(x=w340, y=path "") -> (x != y?=w338:bool)
        n189 = Not(x=w344) -> (.not. x?=w343:bool)
        n190 = case shown="True" w338 {
          tunnel: w343 -> [_ w349]
          tunnel: T14."Multi Measurement" ("Do Measurement") -> [_ w348]
          tunnel: w341 -> [_ w347]
          tunnel: w337 -> [_ w346]
          frame False {
            # "No Workspace Open"
            n191 = One Button Dialog(message="No Workspace Opened") -> ()  [unwired: 1 in, 1 out]
          }
          frame True {
            # "Aquire Image if not Running"
            n192 = case shown="True" w349 {
              tunnel: w348 -> [_ w350]
              tunnel: w347 -> [_ _]
              tunnel: w346 -> [_ _]
              frame False {
              }
              frame True {
                n193 = local write "MeasRunig"(TRUE ("Measurement Running")) -> ()
                n194 = local write "Do Measurement"(w350) -> ()
              }
            }
          }
        }
      }
      event "New MSW": Mouse Up {
        # "Default Name"
        n195 = event-data() -> ()  [unwired: 1 in, 7 out]
        n196 = flat-sequence {
          tunnel: [w372] -> w355
          tunnel: w354 -> [w372]
          frame #0 {
            n197 = local write "MeasRunig"(TRUE ("MeasRunig")) -> ()
          }
        }
        n198 = Get Date/Time In Seconds() -> (seconds since 1Jan1904=w369:timestamp)
        n199 = Format Date/Time String(time format string (%c)="%Y-%m-%d", seconds (now)=w369) -> (date/time string=w367:string)  [unwired: 1 out]
        n200 = Concatenate Strings(w367, ".msw" ("string")) -> (w365:string)
        n201 = call "File Dialog"("start path"=path "X:/MTusers", "prompt"="Create New Workspace", "button label"="Create", "default name"=w365, "error in"=w355, "pattern (all files)"="*.msw", "pattern label"="MT Scan Workspace") -> ("selected path"=w359:path, "cancelled"=w360:bool, "error out"=w358:errorcluster)  [unwired: 5 in, 1 out]
        n202 = case shown="False" w360 {
          tunnel: w359 -> [w378 _]
          tunnel: w358 -> [w384 w386]
          tunnel: [w376 w385] -> w353
          tunnel: w356 -> [w374 _]
          frame False {
            # "Create Empty Workspace"
            n203 = local write "Workspace"(w378) -> ()
            n204 = call "MTS_CreateWriteMSW.vi"("Rewrite"=TRUE, "error in (no error)"=w384, "Workspace Path"=w378) -> ("error out"=w377:errorcluster, "Created"=w381:string, "Comment (dup)"=w380:string, "Files in Workspace (dup)"=w379:T21)  [unwired: 5 in]
            n205 = call "MTS_Workspace.vi"("Workspace"=w378, "Operation"=T18."Set Workspace", "Created in"=w381, "New Comment"=w380, "Files in Workspace in"=w379) -> ("Files in Workspace"=w375:T21)  [unwired: 3 in, 3 out]
            n206 = call "MTS_BuildWSTree.vi"("error in"=w377, "Files in Workspace"=w375, "Tree Refnum"=w374) -> ("error out"=w376:errorcluster)  [unwired: 7 in, 1 out]
          }
          frame True {
            n207 = call <vilib>:"Clear Errors.vi"("error in (no error)"=w386) -> ("error out"=w385:errorcluster)  [unwired: 6 in]
          }
        }
        n208 = flat-sequence {
          tunnel: w353 -> [w370]
          tunnel: [w370] -> w352
          frame #0 {
            n209 = local write "MeasRunig"(FALSE ("MeasRunig")) -> ()
          }
        }
      }
      event "Open MSW": Mouse Up {
        n210 = event-data() -> ()  [unwired: 1 in, 7 out]
        n211 = flat-sequence {
          tunnel: w390 -> [w402]
          tunnel: [w402] -> w389
          frame #0 {
            n212 = local write "MeasRunig"(TRUE ("MeasRunig")) -> ()
          }
        }
        n213 = call "File Dialog2"("start path"=path "X:/MTusers", "prompt"="Create New Workspace", "button label"="Open", "error in"=w389, "pattern (all files)"="*.msw", "pattern label"="MT Scan Workspace") -> ("selected path"=w394:path, "cancelled"=w395:bool, "error out"=w393:errorcluster)  [unwired: 6 in, 1 out]
        n214 = case shown="False" w395 {
          tunnel: w394 -> [w408 _]
          tunnel: w393 -> [w413 w415]
          tunnel: [w406 w414] -> w388
          tunnel: w391 -> [w404 _]
          frame False {
            # "Open Workspace"
            n215 = local write "Workspace"(w408) -> ()
            n216 = call "MTS_ReadMSW.vi"("error in (no error)"=w413, "Workspace Path"=w408) -> ("error out"=w407:errorcluster, "Created"=w411:string, "Comment"=w410:string, "Files in Workspace"=w409:T21)  [unwired: 6 in]
            n217 = call "MTS_Workspace.vi"("Workspace"=w408, "Operation"=T18."Set Workspace", "Created in"=w411, "New Comment"=w410, "Files in Workspace in"=w409) -> ("Files in Workspace"=w405:T21)  [unwired: 3 in, 3 out]
            n218 = call "MTS_BuildWSTree.vi"("error in"=w407, "Files in Workspace"=w405, "Tree Refnum"=w404) -> ("error out"=w406:errorcluster)  [unwired: 7 in, 1 out]
          }
          frame True {
            n219 = call <vilib>:"Clear Errors.vi"("error in (no error)"=w415) -> ("error out"=w414:errorcluster)  [unwired: 6 in]
          }
        }
        n220 = flat-sequence {
          tunnel: w388 -> [w400]
          tunnel: [w400] -> w387
          frame #0 {
            n221 = local write "MeasRunig"(FALSE ("MeasRunig")) -> ()
          }
        }
      }
      event "Image": Mouse Up {
        w418 = 100.0 ("y")
        n222 = event-data() -> ("Coords"=w430:T22, "PlatMods"=w431:T23)  [unwired: 1 in, 5 out]
        n223 = local read "Axis"() -> (w426:enum32{"x-y", "x-z", "y-z"})
        n224 = invoke on="Image" class="IntGraph (strict)" method="Map Coords To XY"("Coords"=w430) -> ("Map Coords To XY"=w427:bool, "XY"=w425:cluster{"X":dbl, "Y":dbl})  [unwired: 6 in, 5 out]
        n225 = Unbundle By Name(w431) -> ("Ctrl"=w428:bool)
        n226 = And(x=w427, y=w428) -> (x .and. y?=w429:bool)
        n227 = Unbundle(w425) -> ("X"=w424:dbl, "Y"=w421:dbl)
        n228 = Multiply(x=w424, y=w418) -> (x*y=w423:dbl)
        n229 = Multiply(x=w421, y=w418) -> (x*y=w420:dbl)
        n230 = Round To Nearest(number=w423) -> (nearest integer value=w422:dbl)
        n231 = Round To Nearest(number=w420) -> (nearest integer value=w419:dbl)
        n232 = Divide(x=w422, y=w418) -> (x/y=w417:dbl)
        n233 = Divide(x=w419, y=w418) -> (x/y=w416:dbl)
        n234 = case shown="True" w429 {
          tunnel: w426 -> [_ w434]
          tunnel: w417 -> [_ w433]
          tunnel: w416 -> [_ w432]
          frame False {
          }
          frame True {
            n235 = case shown="\"x-y\", Default" w434 {
              tunnel: w433 -> [w436 w438 w440]
              tunnel: w432 -> [w435 w437 w439]
              frame "x-y", Default {
                n236 = local write "X-Position"(w436) -> ()
                n237 = local write "Y-Position"(w435) -> ()
              }
              frame "x-z" {
                n238 = local write "X-Position"(w438) -> ()
                n239 = local write "Z-Position"(w437) -> ()
              }
              frame "y-z" {
                n240 = local write "Y-Position"(w440) -> ()
                n241 = local write "Z-Position"(w439) -> ()
              }
            }
          }
        }
      }
      event "WS File Tree": Value Change {
        n242 = event-data() -> ("NewVal"=w446:string)  [unwired: 1 in, 4 out]
        n243 = local read "Workspace"() -> (w443:path)
        n244 = Not Equal?(x=w443, y=path "") -> (x != y?=w444:bool)
        n245 = case shown="True" w444 {
          tunnel: w446 -> [_ w457]
          tunnel: w443 -> [_ w456]
          tunnel: w442 -> [w447 w455]
          tunnel: [w447 w454] -> w441
          frame False {
          }
          frame True {
            n246 = call "MTS_GetFileFromWS.vi"("Tree Label"=w457) -> ("File Header"=w453:T24, "File Found"=w452:bool)  [unwired: 9 in]
            n247 = Unbundle By Name(w453) -> ("File Type"=w451:T19)
            n248 = Equal?(x=w451, y=T19."pt3 File" ("File Type")) -> (x = y?=w449:bool)
            n249 = And(x=w452, y=w449) -> (x .and. y?=w448:bool)
            n250 = case shown="True" w448 {
              tunnel: w453 -> [_ w481]
              tunnel: w456 -> [_ w487]
              tunnel: w455 -> [w458 w482]
              tunnel: [w458 w472] -> w454
              frame False {
              }
              frame True {
                w460 = 1 ("index")
                # "Image Intensity Array"
                n251 = Unbundle By Name(w481) -> ("Measurement Type"=w471:T25, "Pixels"=w469:i32[], "Picture Size"=w466:dbl[], "Upper Left"=w468:T26, "Scan Axis"=w463:enum32{"x-y", "x-z", "y-z"})
                n252 = Unbundle By Name(w481) -> ("File Path"=w486:path)
                n253 = Strip Path(path=w487) -> (stripped path=w485:path)  [unwired: 1 out]
                n254 = Strip Path(path=w486) -> (name=w484:string)  [unwired: 1 out]
                n255 = Index Array(array=w466, index #2=1 ("index")) -> (element #1=w465:dbl, element #2=w464:dbl)  [unwired: 1 in]
                n256 = control-ref of="Image"() -> (w470:refnum<vi>)
                n257 = Build Path(base path=w485, name or relative path=w484) -> (appended path=w483:path)
                n258 = Index Array(array=w469, index #2=w460) -> (element #1=w462:i32, element #2=w461:i32)  [unwired: 1 in]
                n259 = local write "Active pt3"(w483) -> ()
                n260 = call "HT3_Open.vi"("error in"=w482, "File Path"=w483) -> ("error out"=w479:errorcluster, "refnum out"=w478:refnum<file>)  [unwired: 3 in, 5 out]
                n261 = Bundle("Upper Left"=w468, "value"=w465, "value"=w464, "Scan Axis"=w463, "value"=w462, "value"=w461, "index"=w460) -> (w459:T27)  [unwired: 1 in]
                n262 = Initialize Array(0 ("element"), w462, w461) -> (w477:i32[][])
                n263 = case shown="\"Image File\"" w471 {
                  tunnel: w479 -> [w491 w523]
                  tunnel: w478 -> [w498 w522]
                  tunnel: w477 -> [w497 w521]
                  tunnel: [w495 w520] -> w476
                  tunnel: [w494 w519] -> w475
                  tunnel: [w493 w518] -> w474
                  tunnel: [w492 w517] -> w473
                  tunnel: w470 -> [w489 _]
                  tunnel: w459 -> [w488 _]
                  frame "Image File" {
                    n264 = call "MTS_SetGraphScales.vi"("error in (no error)"=w491, "Image Measurent Parameters"=w488, "Image"=w489) -> ("error out"=w490:errorcluster)  [unwired: 8 in]
                    n265 = while {
                      tunnel: w498 -> [w513]
                      shift-right: [FALSE ("Start From Top")] -> _
                      shift-left: TRUE ("Start From Top") -> [w507]
                      shift-right: [w506] -> w492
                      shift-left: w490 -> [w502]
                      tunnel: [w505] -> w493
                      tunnel: [w504] -> w495
                      tunnel: [w503] -> w496
                      tunnel: w497 -> [w501]
                      tunnel: [w500] -> w494
                      stop <- w510 stop-if-true
                      n266 = call "HT3_Read.vi"("Start From Top"=w507, "error in"=w502, "Data count"=10000, "refnum in"=w513) -> ("error out"=w506:errorcluster, "Data out"=w509:u32[], "refnum out"=w505:refnum<file>, "EOF?"=w510:bool)  [unwired: 4 in]
                      n267 = Array Size(array=w509) -> (size(s)=w508:i32)
                      n268 = call "HH_ToImageOffline.vi"("Data In"=w509, "Reset"=w507, "Image Array In"=w501, "Data Count"=w508) -> ("Image Array Out"=w503:i32[][], "Histograms"=w504:i32[][], "Traces"=w500:i32[][])  [unwired: 2 in, 7 out]
                    }
                    n269 = local write "Image"(w496) -> ()
                  }
                  frame "Point Measurement", Default {
                    w524 = TRUE ("Start From Top")
                    n270 = call "HT3_Read.vi"("Start From Top"=w524, "error in"=w523, "Data count"=10000, "refnum in"=w522) -> ("error out"=w517:errorcluster, "Data out"=w515:u32[], "refnum out"=w518:refnum<file>)  [unwired: 4 in, 1 out]
                    n271 = Array Size(array=w515) -> (size(s)=w514:i32)
                    n272 = call "HH_ToImageOffline.vi"("Data In"=w515, "Reset"=w524, "Image Array In"=w521, "Data Count"=w514) -> ("Histograms"=w520:i32[][], "Traces"=w519:i32[][])  [unwired: 2 in, 8 out]
                  }
                }
                n273 = local write "Histogram"(w476) -> ()
                n274 = local write "Trace"(w475) -> ()
                n275 = Close File(refnum=w474, error in=w473) -> (error out=w472:errorcluster)  [unwired: 1 out]
              }
            }
          }
        }
      }
      event "Axis 1 Pixel", "Picture size", "Axis 2 Pixel", "Picture size 2": Value Change {
        w527 = 1000.0 ("y")
        n276 = event-data() -> ()  [unwired: 1 in, 5 out]
        n277 = local read "Picture size 2"() -> (w529:dbl)
        n278 = local read "Picture size"() -> (w533:dbl)
        n279 = local read "Axis 1 Pixel"() -> (w532:u16)
        n280 = local read "Axis 2 Pixel"() -> (w528:u16)
        n281 = Divide(x=w533, y=w532) -> (x/y=w531:dbl)
        n282 = Divide(x=w529, y=w528) -> (x/y=w530:dbl)
        n283 = Multiply(x=w531, y=w527) -> (x*y=→"x":dbl)
        n284 = Multiply(x=w530, y=w527) -> (x*y=→"y":dbl)
      }
      event "Excitation": Mouse Up {
        n285 = event-data() -> ()  [unwired: 1 in, 7 out]
        n286 = local read "MeasRunig"() -> (w535:bool)
        n287 = Not(x=w535) -> (.not. x?=w534:bool)
        n288 = case shown="True" w534 {
          frame False {
          }
          frame True {
            n289 = local read "Excitation"() -> (w541:bool)
            n290 = local read "Detector1"() -> (w540:bool)
            n291 = local read "Detector2"() -> (w539:bool)
            n292 = local read "Detector3"() -> (w537:bool)
            n293 = local read "Detector4"() -> (w536:bool)
            n294 = Not(x=w541) -> (.not. x?=w538:bool)
            n295 = call "PCAN_CompMessage.vi"("Excitation"=w538, "Detector4"=w536, "Detector3"=w537, "Detector2"=w539, "Detector1"=w540) -> ("CAN_Message"=w542:T28)  [unwired: 6 in]
            n296 = call "CAN PCI Write.vi"("CAN_Message"=w542) -> ()  [unwired: 2 in, 1 out]
          }
        }
      }
      event "Detector1": Mouse Up {
        n297 = event-data() -> ()  [unwired: 1 in, 7 out]
        n298 = local read "MeasRunig"() -> (w544:bool)
        n299 = Not(x=w544) -> (.not. x?=w543:bool)
        n300 = case shown="True" w543 {
          frame False {
          }
          frame True {
            n301 = local read "Excitation"() -> (w548:bool)
            n302 = local read "Detector1"() -> (w550:bool)
            n303 = local read "Detector2"() -> (w547:bool)
            n304 = local read "Detector3"() -> (w545:bool)
            n305 = local read "Detector4"() -> (w546:bool)
            n306 = Not(x=w550) -> (.not. x?=w549:bool)
            n307 = call "PCAN_CompMessage.vi"("Excitation"=w548, "Detector4"=w546, "Detector3"=w545, "Detector2"=w547, "Detector1"=w549) -> ("CAN_Message"=w551:T28)  [unwired: 6 in]
            n308 = call "CAN PCI Write.vi"("CAN_Message"=w551) -> ()  [unwired: 2 in, 1 out]
          }
        }
      }
      event "Detector2": Mouse Up {
        n309 = event-data() -> ()  [unwired: 1 in, 7 out]
        n310 = local read "MeasRunig"() -> (w553:bool)
        n311 = Not(x=w553) -> (.not. x?=w552:bool)
        n312 = case shown="True" w552 {
          frame False {
          }
          frame True {
            n313 = local read "Excitation"() -> (w559:bool)
            n314 = local read "Detector1"() -> (w558:bool)
            n315 = local read "Detector2"() -> (w556:bool)
            n316 = local read "Detector3"() -> (w554:bool)
            n317 = local read "Detector4"() -> (w555:bool)
            n318 = Not(x=w556) -> (.not. x?=w557:bool)
            n319 = call "PCAN_CompMessage.vi"("Excitation"=w559, "Detector4"=w555, "Detector3"=w554, "Detector2"=w557, "Detector1"=w558) -> ("CAN_Message"=w560:T28)  [unwired: 6 in]
            n320 = call "CAN PCI Write.vi"("CAN_Message"=w560) -> ()  [unwired: 2 in, 1 out]
          }
        }
      }
      event "Detector3": Mouse Up {
        n321 = event-data() -> ()  [unwired: 1 in, 7 out]
        n322 = local read "MeasRunig"() -> (w562:bool)
        n323 = Not(x=w562) -> (.not. x?=w561:bool)
        n324 = case shown="True" w561 {
          frame False {
          }
          frame True {
            n325 = local read "Excitation"() -> (w568:bool)
            n326 = local read "Detector1"() -> (w567:bool)
            n327 = local read "Detector2"() -> (w563:bool)
            n328 = local read "Detector3"() -> (w565:bool)
            n329 = local read "Detector4"() -> (w566:bool)
            n330 = Not(x=w565) -> (.not. x?=w564:bool)
            n331 = call "PCAN_CompMessage.vi"("Excitation"=w568, "Detector4"=w566, "Detector3"=w564, "Detector2"=w563, "Detector1"=w567) -> ("CAN_Message"=w569:T28)  [unwired: 6 in]
            n332 = call "CAN PCI Write.vi"("CAN_Message"=w569) -> ()  [unwired: 2 in, 1 out]
          }
        }
      }
      event "Detector4": Mouse Up {
        n333 = event-data() -> ()  [unwired: 1 in, 7 out]
        n334 = local read "MeasRunig"() -> (w571:bool)
        n335 = Not(x=w571) -> (.not. x?=w570:bool)
        n336 = case shown="True" w570 {
          frame False {
          }
          frame True {
            n337 = local read "Excitation"() -> (w577:bool)
            n338 = local read "Detector1"() -> (w576:bool)
            n339 = local read "Detector2"() -> (w575:bool)
            n340 = local read "Detector3"() -> (w572:bool)
            n341 = local read "Detector4"() -> (w574:bool)
            n342 = Not(x=w574) -> (.not. x?=w573:bool)
            n343 = call "PCAN_CompMessage.vi"("Excitation"=w577, "Detector4"=w573, "Detector3"=w572, "Detector2"=w575, "Detector1"=w576) -> ("CAN_Message"=w578:T28)  [unwired: 6 in]
            n344 = call "CAN PCI Write.vi"("CAN_Message"=w578) -> ()  [unwired: 2 in, 1 out]
          }
        }
      }
    }
    n345 = flat-sequence {
      tunnel: [w135] -> w132
      tunnel: w131 -> [w135]
      frame #0 {
      }
    }
    n346 = local read "Global Stop"() -> (w130:bool)
  }
  n347 = while {
    shift-right: [w586] -> w29
    shift-left: w31 -> [w581]
    tunnel: w8 -> [w594]
    tunnel: [w593] -> w35
    shift-right: [w588] -> w15
    shift-left: w32 -> [w595]
    tunnel: w30 -> [w587]
    shift-right: [w584] -> w13
    shift-left: w12 -> [w583]
    tunnel: w1 -> [w579]
    stop <- w591 stop-if-true
    n348 = case shown="No Error" w581 {
      selector: w581 -> [w608 w1491]
      tunnel: w595 -> [w622 w1489]
      tunnel: w594 -> [w621 w1490]
      tunnel: [w620 w1490] -> w593
      tunnel: [w619 TRUE ("Global Stop")] -> w590
      tunnel: [w615 w1489] -> w589
      tunnel: w587 -> [w614 _]
      tunnel: [w613 w1491] -> w586
      tunnel: [w611 w1488] -> w584
      tunnel: w583 -> [w610 w1488]
      tunnel: [w609 T5."No Measurement" ("Do Measurement")] -> w582
      tunnel: [w606 FALSE] -> w580
      tunnel: w579 -> [w605 _]
      frame No Error {
        # "Wait for Start"
        n349 = while {
          shift-right: [w1484] -> w616
          shift-left: w622 -> [w1484]
          tunnel: [w1481] -> w618
          tunnel: [w1480] -> w617
          tunnel: [w1479] -> w612
          stop <- w1485 stop-if-true
          w1479 = FALSE ("FiFo Overrun")
          n350 = local read "Do Measurement"() -> (w1481:T5)
          n351 = local read "Global Stop"() -> (w1480:bool)
          n352 = Wait (ms)(milliseconds to wait=u32 100) -> ()  [unwired: 1 out]
          n353 = local write "Stop Measurement"(w1479) -> ()
          n354 = Greater Than 0?(x=w1481) -> (x > 0?=w1483:bool)
          n355 = Or(x=w1483, y=w1480) -> (x .or. y?=w1485:bool)
        }
        n356 = Build Array("X-Axis Offset", "Y-Axis Offset", "Z-Axis Offset") -> (w596:dbl[])
        n357 = control-ref of="WS File Tree"() -> (w607:refnum<vi>)
        n358 = local write "FiFo Overrun"(w612) -> ()
        n359 = Build Array("X-Axis Points", "Y-Axis Points", "Z-Axis Points") -> (w600:u16[])
        n360 = case shown="\"Aquire Image\", \"Aquire Line Scan\"" w618 {
          selector: w618 -> [_ w640 w911 _ _ _ _ _]
          tunnel: w608 -> [w628 w705 w959 w1128 w1286 w1302 w1378 w1447]
          tunnel: w621 -> [w629 w704 w925 w1129 w1287 w1298 w1374 w1446]
          tunnel: [w629 w676 w914 w1059 w1279 w1298 w1374 w1446] -> w620
          tunnel: [w628 w682 w949 w1118 w1280 w1301 w1377 w1447] -> w613
          tunnel: [w627 FALSE ("Global Stop") FALSE ("Global Stop") FALSE ("Global Stop") FALSE ("Global Stop") FALSE ("Global Stop") FALSE ("Global Stop") FALSE ("Global Stop")] -> w619
          tunnel: w617 -> [w627 _ _ _ _ _ _ _]
          tunnel: w616 -> [w626 w671 w943 w1075 w1278 w1300 w1376 w1442]
          tunnel: [w626 w683 w950 w1119 w1278 w1300 w1376 w1438] -> w615
          tunnel: w614 -> [_ w701 w956 w1107 _ _ _ _]
          tunnel: w610 -> [w625 w655 w912 w1122 w1276 w1290 w1362 w1431]
          tunnel: [w625 w655 w912 w1122 w1276 w1290 w1361 w1430] -> w611
          tunnel: [T5."No Measurement" ("Do Measurement") T5."No Measurement" ("Do Measurement") w909 T5."No Measurement" ("Do Measurement") T5."No Measurement" ("Do Measurement") T5."No Measurement" ("Do Measurement") T5."No Measurement" ("Do Measurement") w1437] -> w609
          tunnel: w607 -> [_ _ w893 w1062 _ _ _ _]
          tunnel: [FALSE FALSE w879 FALSE FALSE FALSE FALSE FALSE] -> w606
          tunnel: w605 -> [_ w649 _ _ _ _ _ _]
          tunnel: T5."Aquire Line Scan" ("Do Measurement") -> [_ w639 _ _ _ _ _ _]
          tunnel: w600 -> [_ _ _ w1061 _ _ _ _]
          tunnel: w596 -> [_ _ _ w1060 _ _ _ _]
          frame "No Measurement", Default {
          }
          frame "Aquire Image", "Aquire Line Scan" {
            w653 = 32768 ("dimension size")
            # "Line Scan"
            # "TODO:\n- FIFO Read Flag Buffer Half Full?\n- auto square pixels"
            # "Image Intensity Array"
            n361 = control-ref of="Image"() -> (w660:refnum<vi>)
            n362 = Equal?(x=w640, y=w639) -> (x = y?=w635:bool)
            n363 = Bundle("X-Position"="X-Position", "Y-Position"="Y-Position", "Z-Position"="Z-Position") -> (w648:T31)  [unwired: 1 in]
            n364 = Cluster To Array(cluster=w648) -> (array=w703:dbl[])
            n365 = case shown="False" w635 {
              tunnel: "Picture size" -> [w723 _]
              tunnel: "Picture size 2" -> [w722 _]
              tunnel: [T29."Image File" ("Measurement Type") T29."Line Scan" ("Measurement Type")] -> w656
              tunnel: w649 -> [w720 w734]
              tunnel: w648 -> [w717 w727]
              tunnel: "Scanner Divider" -> [w716 _]
              tunnel: "Axis" -> [w715 _]
              tunnel: "Axis 1 Pixel" -> [w714 _]
              tunnel: "Axis 2 Pixel" -> [w713 _]
              tunnel: [w712 w729] -> w631
              frame False {
                n366 = call "PI_Scanner_In_Range.vi"("Picture size"=w723, "Picture size 2"=w722, "Upper Left"=w717, "Axis"=w715) -> ("Picture size out"=w719:dbl, "Picture size out 2"=w718:dbl)  [unwired: 14 in]
                n367 = Bundle By Name(cluster=w720, "Position"=w717, "Picture Size Axis 1"=w719, "Picture Size Axis 2"=w718, "Axis"=w715, "Axis 1 Pixels"=w714, "Axis 2 Pixels"=w713, "Scanner Divider"=w716) -> (w712:T6)
                n368 = local write "Picture size"(w719) -> ()
                n369 = local write "Picture size 2"(w718) -> ()
              }
              frame True {
                # "Line Scan"
                n370 = call "PI_ScannerLine_In_Range.vi"("Line Width"="Line Width", "Line Scan Axis"="Line Scan Axis", "Starting Point"=w727) -> ("Line Width out"=w724:dbl)  [unwired: 16 in]
                n371 = Bundle By Name(cluster=w734, "Position"=w727, "Picture Size Axis 1"=w724, "Picture Size Axis 2"=1.0, "Axis"="Line Scan Axis", "Axis 1 Pixels"="Line Points", "Axis 2 Pixels"=u16 1, "Scanner Divider"="Line Scanner Divider") -> (w729:T6)
                n372 = local write "Line Width"(w724) -> ()
              }
            }
            n373 = call "PI_MoveTo.vi"("System no."=w704, "Target position"=w703, "error in"=w705, "Move"=TRUE) -> ("System no. (dup)"=w688:i32, "error out"=w659:errorcluster)  [unwired: 13 in, 1 out]
            n374 = local read "Workspace"() -> (w670:path)
            n375 = control-ref of="WS File Tree"() -> (w664:refnum<vi>)
            n376 = call "MTS_SetGraphScales.vi"("error in (no error)"=w659, "Image Measurent Parameters"=w631, "Image"=w660) -> ("error out"=w657:errorcluster)  [unwired: 8 in]
            n377 = call "PI_Image_Scanner_Prepare_Dlg.vi"("System no."=w688, "Image Measurent Parameters"=w631, "Line Scan"=w635, "error in"=w657, "Learning loop"="Learning loop") -> ("System no. (dup)"=w687:i32, "Measurement time [s]"=w686:dbl, "error out"=w689:errorcluster)  [unwired: 8 in]
            n378 = Index Array(array=w701) -> (element=w700:T32)  [unwired: 1 in]
            n379 = call "HH_Set.vi"("Device List"=w701, "CFD Settings"="CFD Settings", "error in (no error)"=w689) -> ("ht3 header out"=w673:T33, "Sync Rate"=w691:i32, "error out"=w675:errorcluster)  [unwired: 8 in, 2 out]
            n380 = Initialize Array(0 ("element"), "Axis 1 Pixel", "Axis 2 Pixel") -> (w692:i32[][])
            n381 = Unbundle By Name(w700) -> ("Dev"=w697:i32)
            n382 = call "MTS_PreapareImage.vi"("WS File Tree"=w664, "Workspace"=w670, "Measurement Type"=w656, "Image Measurent Parameters"=w631, "error in"=w671) -> ("File Name (dup)"=w643:path, "File No"=→"Last Image File No":i32, "Image Header"=w641:T34, "Comment"=w642:string, "error out"=w665:errorcluster)  [unwired: 6 in]
            n383 = call "MTS_CalcMeasTime.vi"("Image Measurent Parameters"=w631, "ht3 header in"=w673, "Measurement time [s]"=w686, "Count Rate"=w691) -> ("ht3 header out"=w672:T33, "Corrected Measurement time [s]"=→"Measure. time [s]":i32, "Calc Acq. Time (ms)"=w638:i32, "Overflow Interv. Time (s)"=w694:dbl, "Pixel Time (Laser Pulses)"=w690:i32)  [unwired: 7 in]
            n384 = Multiply(x="Line Time (s)", y=1000 ("x")) -> (x*y=w634:i32)
            n385 = Select(t=w634, s=w635, f=w638) -> (s? t:f=w637:i32)
            n386 = call "HT3_Create.vi"("Image Header in"=w641, "Save pt3"="Save Files", "Measurement Type"=w656, "error in"=w675, "Comment"=w642, "ht3 Header in"=w672, "File Path"=w643) -> ("error out"=w674:errorcluster, "FileHeaderPos"=w652:T35, "refnum out"=w669:refnum<file>)  [unwired: 2 in]
            n387 = local write "Active pt3"(w643) -> ()
            n388 = call "HH_Start.vi"("Device Index"=w697, "Acq. Time"=w637, "error in (no error)"=w674) -> ("error out"=w698:errorcluster)  [unwired: 11 in, 1 out]
            n389 = Unbundle By Name(w698) -> ("status"=w699:bool)
            n390 = Unbundle By Name(w631) -> ("Axis"=w636:i32)
            n391 = Initialize Array(u32 0, w653) -> (w680:u32[])
            n392 = Not(x=w699) -> (.not. x?=w696:bool)
            n393 = case shown="True" w696 {
              tunnel: [w796 w825] -> w684
              tunnel: [w798 w817] -> w677
              tunnel: w687 -> [w798 w814]
              tunnel: w698 -> [w797 w815]
              tunnel: w665 -> [w799 w823]
              tunnel: [w799 w822] -> w685
              tunnel: w697 -> [w795 w824]
              tunnel: w694 -> [_ w804]
              tunnel: w692 -> [_ w819]
              tunnel: w690 -> [_ w818]
              tunnel: w636 -> [_ w813]
              tunnel: w680 -> [_ w812]
              tunnel: w653 -> [_ w811]
              tunnel: [w794 w810] -> w679
              tunnel: [w794 w809] -> w678
              tunnel: w669 -> [w793 w808]
              tunnel: [w793 w807] -> w668
              tunnel: [0 ("Num Records Total") w806] -> w667
              tunnel: [0.0 w803] -> w666
              tunnel: [u64[] [] ("Histograms") w802] -> w663
              tunnel: w635 -> [_ w801]
              tunnel: w635 -> [_ w800]
              frame False {
                w794 = FALSE ("Stop Measurement")
                n394 = call "HH_Stop.vi"("Device Index"=w795, "error in (no error)"=w797) -> ("error out"=w796:errorcluster)  [unwired: 12 in, 1 out]
              }
              frame True {
                # "Overflow Interv. Time (s)"
                # "No Error"
                n395 = call "PI_Start_Wave_Gen.vi"("System no."=w814, "error in"=w815, "Axis"=w813, "Line Scan"=w800) -> ("System no. (dup)"=w817:i32, "error out"=w816:errorcluster)  [unwired: 10 in]
                n396 = while {
                  tunnel: w824 -> [w854]
                  tunnel: w812 -> [w853]
                  tunnel: w811 -> [w852]
                  shift-right: [w838] -> w821
                  shift-left: w816 -> [w855]
                  shift-right: [w851] -> w822
                  shift-left: w823 -> [w851]
                  shift-right: [FALSE ("Reset")] -> _
                  shift-left: TRUE ("Reset") -> [w847]
                  tunnel: w819 -> [w844]
                  tunnel: w818 -> [w840]
                  tunnel: [w841] -> w810
                  tunnel: [w831] -> w809
                  tunnel: w808 -> [w835]
                  tunnel: [w834] -> w807
                  tunnel: [w833] -> w806
                  tunnel: [w832] -> w805
                  tunnel: [w827] -> w802
                  tunnel: w801 -> [w826]
                  stop <- w850 stop-if-true
                  # "Is Line Scan?"
                  n397 = call "HH_FIFORead.vi"("Device Index"=w854, "Buffer In"=w853, "Count"=w852, "error in (no error)"=w855) -> ("OK"=w842:bool, "Buffer Out"=w836:u32[], "Data Count"=w837:i32, "FiFo Overrun"=w841:bool, "error out"=w839:errorcluster)  [unwired: 7 in]
                  n398 = local write "FiFo Overrun"(w841) -> ()
                  n399 = local read "Global Stop"() -> (w829:bool)
                  n400 = Wait (ms)(milliseconds to wait=u32 10) -> ()  [unwired: 1 out]
                  n401 = Unbundle(w839) -> ("status"=w849:bool)  [unwired: 2 out]
                  n402 = case shown="True" w826 {
                    tunnel: w847 -> [w866 w870]
                    tunnel: [w865 w875] -> w845
                    tunnel: w844 -> [w864 w867]
                    tunnel: [w863 w867] -> w843
                    tunnel: w840 -> [w862 _]
                    tunnel: w837 -> [w861 w868]
                    tunnel: w836 -> [w860 w869]
                    tunnel: [w859 w872] -> w833
                    tunnel: [w858 w871] -> w832
                    tunnel: [w857 w874] -> w828
                    tunnel: [w856 w873] -> w827
                    frame False {
                      n403 = call "HH_ToImage.vi"("Data In"=w860, "Reset"=w866, "Image Array In"=w864, "Data Count"=w861, "Pixel Time (Laser Pulses)"=w862) -> ("Image Array Out"=w863:i32[][], "Histograms"=w857:i32[][], "Total Photon Count"=w856:u64[], "Total Oveflow Count"=w858:u64, "Num Records Total"=w859:i64, "Traces"=w865:i32[][])  [unwired: 4 in, 1 out]
                    }
                    frame True {
                      n404 = call "HH_TraceAndHisto.vi"("Data In"=w869, "Reset"=w870, "Data Count"=w868) -> ("Histograms"=w874:i32[][], "Total Photon Count"=w873:u64[], "Total Oveflow Count"=w871:u64, "Num Records Total"=w872:i64, "Traces"=w875:i32[][])  [unwired: 8 in]
                    }
                  }
                  "Histogram" <- w828
                  "Trace" <- w845
                  "Image" <- w843
                  n405 = local read "Stop Measurement"() -> (w830:bool)
                  n406 = call "HT3_Write.vi"("error in"=w839, "Data Count"=w837, "Data in"=w836, "refnum in"=w835) -> ("error out"=w838:errorcluster, "refnum out"=w834:refnum<file>)  [unwired: 6 in]
                  n407 = Compound Arithmetic op=OR(invert w842, w849, w829, w830) -> (w850:bool)
                  n408 = Or(x=w830, y=w829) -> (x .or. y?=w831:bool)
                }
                n409 = Multiply(x=w804, y=w805) -> (x*y=w803:dbl)
                n410 = call "HH_Stop.vi"("Device Index"=w824, "error in (no error)"=w821) -> ("error out"=w825:errorcluster)  [unwired: 12 in, 1 out]
              }
            }
            n411 = control-ref of="WS File Tree"() -> (w661:refnum<vi>)
            n412 = flat-sequence {
              tunnel: w685 -> [w765]
              tunnel: w684 -> [w762]
              tunnel: [w765] -> w683
              tunnel: [w741] -> w682
              tunnel: w679 -> [w764]
              tunnel: w678 -> [w752]
              tunnel: w677 -> [w761]
              tunnel: [w760] -> w676
              tunnel: w668 -> [w758]
              tunnel: w667 -> [w757]
              tunnel: w666 -> [w750]
              tunnel: w663 -> [w751]
              tunnel: "Save Files" -> [w740]
              tunnel: w643 -> [w739]
              tunnel: w661 -> [w738]
              tunnel: w652 -> [w737]
              tunnel: w635 -> [w736]
              tunnel: w635 -> [w735]
              frame #0 {
                # "Is Line Scan?"
                # "Count Rate (per s)"
                # "Stop WaveGen\nif Aborted"
                # "Finish after Aquire Image"
                n413 = Or(x=w752, y=w764) -> (x .or. y?=w763:bool)
                n414 = case shown="True" w763 {
                  tunnel: w762 -> [w774 w789]
                  tunnel: w761 -> [w772 w788]
                  tunnel: [w771 w787] -> w760
                  tunnel: [w773 w786] -> w759
                  tunnel: [enum16{"timeover", "manual", "overflow"}."timeover" ("Stop Reason") w784] -> w753
                  tunnel: w752 -> [_ w782]
                  tunnel: w735 -> [w770 _]
                  frame False {
                    n415 = case shown="True" w770 {
                      tunnel: w774 -> [w776 w781]
                      tunnel: [w776 w780] -> w773
                      tunnel: w772 -> [w777 w779]
                      tunnel: [w777 w778] -> w771
                      frame False {
                      }
                      frame True {
                        n416 = call "PI_Stop_Wave_Gen.vi"("System no."=w779, "error in"=w781) -> ("System no. (dup)"=w778:i32, "error out"=w780:errorcluster)  [unwired: 12 in]
                      }
                    }
                  }
                  frame True {
                    n417 = call "PI_Stop_Wave_Gen.vi"("System no."=w788, "error in"=w789) -> ("System no. (dup)"=w787:i32, "error out"=w786:errorcluster)  [unwired: 12 in]
                    n418 = Select(t=enum16{"timeover", "manual", "overflow"}."manual" ("Stop Reason"), s=w782, f=enum16{"timeover", "manual", "overflow"}."overflow" ("Stop Reason")) -> (s? t:f=w784:enum16{"timeover", "manual", "overflow"})
                  }
                }
                n419 = Multiply(x=w750, y=1000.0) -> (x*y=w755:dbl)
                n420 = Divide(x=w751, y=w750) -> (x/y=w749:dbl[])
                n421 = case shown="False" w736 {
                  frame True {
                    n422 = property on="Line Scan" class="Bool"("BoolText.Text"="Start Line Scan" ("Caption.Text"), "BoolText.TextColor"=u32 0 ("Boolean Text.Colors:FG Color")) -> ()  [unwired: 2 in, 2 out]
                  }
                  frame False {
                    n423 = property on="Aquire Image" class="Bool"("BoolText.Text"="Aquire Image" ("Caption.Text"), "BoolText.TextColor"=u32 0 ("Boolean Text.Colors:FG Color")) -> ()  [unwired: 2 in, 2 out]
                  }
                }
                n424 = To Long Integer(number=w755) -> (32bit integer=w754:i32)
                n425 = To Long Integer(number=w749) -> (32bit integer=w748:i32[])
                n426 = Index Array(array=w748, index #1=0 ("index"), index #2=1 ("index")) -> (element #1=w745:i32, element #2=w744:i32)
                n427 = local read "Image"() -> (w743:i32[][])
                n428 = call "HT3_Finish.vi"("Input 1 Rate"=w744, "FileHeaderPos"=w737, "Input 0 Rate"=w745, "Stop Reason"=w753, "error in"=w759, "Num Records"=w757, "Stop After (ms)"=w754, "refnum in"=w758) -> ("error out"=w742:errorcluster)  [unwired: 3 in]
                n429 = call "MTS_SaveImagePng.vi"("Save .png"=w740, "Tree Refnum"=w738, ".pt3 File Name"=w739, "error in"=w742, "Image"=w743) -> ("error out"=w741:errorcluster)  [unwired: 6 in]
              }
            }
          }
          frame "Point Measurement", "Auto Point" {
            w890 = 32768 ("dimension size")
            n430 = local read "Workspace"() -> (w941:path)
            n431 = local read "X-Position"() -> (w928:dbl)
            n432 = local read "Y-Position"() -> (w927:dbl)
            n433 = local read "Z-Position"() -> (w926:dbl)
            n434 = local read "Pattern"() -> (w895:dbl[][])
            n435 = local read "NxtAutMesPoint"() -> (w894:i32)
            n436 = local read "Last Image File No"() -> (w900:i32)
            n437 = Index Array(array=w956) -> (element=w955:T32)  [unwired: 1 in]
            n438 = Bundle("X-Position"=w928, "Y-Position"=w927, "Z-Position"=w926) -> (w897:T31)  [unwired: 1 in]
            n439 = Equal?(x=w911, y=T16."Auto Point" ("Do Measurement")) -> (x = y?=w881:bool)
            n440 = local read "CFD Settings"() -> (w878:T4)
            n441 = Unbundle By Name(w955) -> ("Dev"=w915:i32)
            n442 = call "MTS_AutoPointCords.vi"("Is Auto Point"=w881, "Cords In"=w897, "Next Auto Measure Point"=w894, "Pattern"=w895) -> ("Cords"=w896:T31)  [unwired: 7 in]
            n443 = Cluster To Array(cluster=w896) -> (array=w958:dbl[])
            n444 = Select(t="Auto Measurement Time (ms)", s=w881, f="Measurement Time (s)") -> (s? t:f=w888:i32)
            n445 = Multiply(x=w888, y=1000) -> (x*y=w887:i32)
            n446 = call "PI_MoveTo.vi"("System no."=w925, "Target position"=w958, "error in"=w959, "Move"=TRUE) -> ("System no. (dup)"=w914:i32, "error out"=w929:errorcluster)  [unwired: 13 in, 1 out]
            n447 = Select(t="AutoPoint" ("Measurement Type"), s=w881, f="Point" ("Measurement Type")) -> (s? t:f=w903:string)
            n448 = Select(t=T30."Auto Point" ("Measurement Type"), s=w881, f=T30."Point Measurement" ("Measurement Type")) -> (s? t:f=w904:T30)
            n449 = Select(t=w900, s=w881, f=-1) -> (s? t:f=w898:i32)
            n450 = call "MTS_GenFileComment.vi"("Parent File No"=w898, "Measurement Type"=w904, "error in"=w943, "Upper Left"=w896) -> ("error out"=w940:errorcluster, "Image Info"=w930:T36, "Comment"=w942:string)  [unwired: 4 in, 1 out]
            n451 = call "HH_Set.vi"("Device List"=w956, "CFD Settings"=w878, "error in (no error)"=w929) -> ("ht3 header out"=w921:T33, "Sync Rate"=w922:i32, "error out"=w917:errorcluster)  [unwired: 8 in, 2 out]
            n452 = Bundle By Name(cluster=w921, "AcquisitionTime (ms)"=w887) -> (w920:T33)
            n453 = And(x=w881, y="Autopoint-Auto Z") -> (x .and. y?=w891:bool)
            n454 = Reciprocal(x=w922) -> (1/x=w924:dbl)
            n455 = call "MTS_GetNextFileName.vi"("error in (no error)"=w940, "File Type"="ht3", "Measurement Type"=w903, "Workspace"=w941) -> ("error out"=w934:errorcluster, "Next File Name"=w933:path)  [unwired: 6 in]
            n456 = Scale By Power Of 2(n=16, x=w924) -> (x*2^n=w913:dbl)
            n457 = case shown="True" w891 {
              tunnel: w917 -> [w965 w973]
              tunnel: [w965 w972] -> w916
              tunnel: w915 -> [_ w971]
              tunnel: w914 -> [_ w970]
              tunnel: w913 -> [_ w969]
              tunnel: w896 -> [_ w968]
              frame False {
              }
              frame True {
                # "Auto Z"
                n458 = call "MTS_AutoZPos.vi"("PH Dev"=w971, "OFlow Interv [s]"=w969, "PI System no."=w970, "error in"=w973, "Start Point"=w968) -> ("New Z"=w967:dbl, "Counts"=→"Counts":u32[], "error out"=w972:errorcluster)  [unwired: 8 in]
                n459 = local write "Z-Position"(w967) -> ()
              }
            }
            n460 = call "MTS_AddFileToWorkspace.vi"("File Name"=w933, "File Type"=T19."pt3 File", "Measurement Type"=w904, "File Info"=w930, "error in (no error)"=w934, "Parent"=w898, "Tree Refnum"=w893) -> ("File Name (dup)"=w931:path, "error out"=w932:errorcluster)  [unwired: 6 in, 1 out]
            n461 = call "HT3_Create.vi"("error in"=w916, "Comment"=w942, "ht3 Header in"=w920, "File Path"=w931) -> ("error out"=w944:errorcluster, "FileHeaderPos"=w889:T35, "refnum out"=w938:refnum<file>)  [unwired: 5 in]
            n462 = And(x="Auto Shutter Control", y=w881) -> (x .and. y?=w882:bool)
            n463 = call "HH_Start.vi"("Device Index"=w915, "Acq. Time"=w887, "error in (no error)"=w944) -> ("error out"=w885:errorcluster)  [unwired: 11 in, 1 out]
            n464 = Initialize Array(u32 0, w890) -> (w947:u32[])
            n465 = Unbundle By Name(w885) -> ("status"=w954:bool)
            n466 = case shown="True" w882 {
              tunnel: w885 -> [w961 w964]
              tunnel: [w961 w964] -> w884
              frame False {
              }
              frame True {
                w962 = TRUE ("Auto Shutter Control")
                n467 = call "PCAN_CompMessage.vi"("Excitation"=w962, "Detector4"=w962, "Detector3"=w962, "Detector2"=w962, "Detector1"=w962) -> ("CAN_Message"=w963:T28)  [unwired: 6 in]
                n468 = call "CAN PCI Write.vi"("CAN_Message"=w963) -> ()  [unwired: 2 in, 1 out]
              }
            }
            n469 = Not(x=w954) -> (.not. x?=w953:bool)
            n470 = case shown="True" w953 {
              tunnel: [w1011 w1031] -> w951
              tunnel: w884 -> [w1012 w1015]
              tunnel: w932 -> [w1013 w1029]
              tunnel: [w1013 w1028] -> w952
              tunnel: w915 -> [w1010 w1030]
              tunnel: w913 -> [_ w1017]
              tunnel: w947 -> [_ w1025]
              tunnel: w890 -> [_ w1024]
              tunnel: [w1009 w1023] -> w946
              tunnel: [w1009 w1022] -> w945
              tunnel: w938 -> [w1008 w1021]
              tunnel: [w1008 w1020] -> w937
              tunnel: [i64 0 ("Num Records Total") w1019] -> w936
              tunnel: [0.0 w1016] -> w935
              tunnel: [u64[] [] ("Total Photon Count") w1014] -> w919
              frame False {
                w1009 = FALSE ("Stop Measurement")
                n471 = call "HH_Stop.vi"("Device Index"=w1010, "error in (no error)"=w1012) -> ("error out"=w1011:errorcluster)  [unwired: 12 in, 1 out]
              }
              frame True {
                # "Overflow Interv. Time (s)"
                # "No Error"
                n472 = while {
                  tunnel: w1030 -> [w1056]
                  tunnel: w1025 -> [w1055]
                  tunnel: w1024 -> [w1054]
                  shift-right: [w1044] -> w1027
                  shift-left: w1015 -> [w1057]
                  shift-right: [w1053] -> w1028
                  shift-left: w1029 -> [w1053]
                  shift-right: [FALSE ("Reset")] -> _
                  shift-left: TRUE ("Reset") -> [w1049]
                  tunnel: [w1046] -> w1023
                  tunnel: [w1037] -> w1022
                  tunnel: w1021 -> [w1041]
                  tunnel: [w1040] -> w1020
                  tunnel: [w1039] -> w1019
                  tunnel: [w1038] -> w1018
                  tunnel: [w1032] -> w1014
                  stop <- w1052 stop-if-true
                  n473 = call "HH_FIFORead.vi"("Device Index"=w1056, "Buffer In"=w1055, "Count"=w1054, "error in (no error)"=w1057) -> ("OK"=w1047:bool, "Buffer Out"=w1042:u32[], "Data Count"=w1043:i32, "FiFo Overrun"=w1046:bool, "error out"=w1045:errorcluster)  [unwired: 7 in]
                  n474 = local write "FiFo Overrun"(w1046) -> ()
                  n475 = local read "Global Stop"() -> (w1035:bool)
                  n476 = Wait (ms)(milliseconds to wait=u32 10) -> ()  [unwired: 1 out]
                  n477 = Unbundle(w1045) -> ("status"=w1051:bool)  [unwired: 2 out]
                  n478 = call "HH_TraceAndHisto.vi"("Data In"=w1042, "Reset"=w1049, "Data Count"=w1043) -> ("Histograms"=w1034:i32[][], "Total Photon Count"=w1032:u64[], "Total Oveflow Count"=w1038:u64, "Num Records Total"=w1039:i64, "Traces"=w1033:i32[][])  [unwired: 8 in]
                  n479 = local read "Stop Measurement"() -> (w1036:bool)
                  n480 = call "HT3_Write.vi"("error in"=w1045, "Data Count"=w1043, "Data in"=w1042, "refnum in"=w1041) -> ("error out"=w1044:errorcluster, "refnum out"=w1040:refnum<file>)  [unwired: 6 in]
                  n481 = local write "Histogram"(w1034) -> ()
                  n482 = local write "Trace"(w1033) -> ()
                  n483 = Compound Arithmetic op=OR(invert w1047, w1051, w1035, w1036) -> (w1052:bool)
                  n484 = Or(x=w1036, y=w1035) -> (x .or. y?=w1037:bool)
                }
                n485 = Multiply(x=w1017, y=w1018) -> (x*y=w1016:dbl)
                n486 = call "HH_Stop.vi"("Device Index"=w1030, "error in (no error)"=w1027) -> ("error out"=w1031:errorcluster)  [unwired: 12 in, 1 out]
              }
            }
            n487 = flat-sequence {
              tunnel: w952 -> [w997]
              tunnel: w951 -> [w993]
              tunnel: [w997] -> w950
              tunnel: [w990] -> w949
              tunnel: w946 -> [w995]
              tunnel: w945 -> [w983]
              tunnel: w937 -> [w989]
              tunnel: w936 -> [w988]
              tunnel: w935 -> [w978]
              tunnel: w919 -> [w977]
              tunnel: w889 -> [w974]
              frame #0 {
                # "Finish after Measurement"
                n488 = Or(x=w983, y=w995) -> (x .or. y?=w994:bool)
                n489 = case shown="True" w994 {
                  tunnel: w993 -> [w999 w1000]
                  tunnel: [w999 w1000] -> w991
                  tunnel: [enum16{"timeover", "manual", "overflow"}."timeover" ("Stop Reason") w1003] -> w984
                  tunnel: w983 -> [_ w1001]
                  frame False {
                  }
                  frame True {
                    n490 = Select(t=enum16{"timeover", "manual", "overflow"}."manual" ("Stop Reason"), s=w1001, f=enum16{"timeover", "manual", "overflow"}."overflow" ("Stop Reason")) -> (s? t:f=w1003:enum16{"timeover", "manual", "overflow"})
                  }
                }
                n491 = Multiply(x=w978, y=1000.0) -> (x*y=w986:dbl)
                n492 = Divide(x=w977, y=w978) -> (x/y=w979:dbl[])
                n493 = To Long Integer(number=w986) -> (32bit integer=w985:i32)
                n494 = To Long Integer(number=w979) -> (32bit integer=w980:i32[])
                n495 = property on="Point Measurement" class="Bool"("BoolText.Text"="Point Measurement" ("Caption.Text"), "BoolText.TextColor"=u32 0 ("Boolean Text.Colors:FG Color")) -> ()  [unwired: 2 in, 2 out]
                n496 = Index Array(array=w980, index #1=0 ("index"), index #2=1 ("index")) -> (element #1=w976:i32, element #2=w975:i32)
                n497 = call "HT3_Finish.vi"("Input 1 Rate"=w975, "FileHeaderPos"=w974, "Input 0 Rate"=w976, "Stop Reason"=w984, "error in"=w991, "Num Records"=w988, "Stop After (ms)"=w985, "refnum in"=w989) -> ("error out"=w990:errorcluster)  [unwired: 3 in]
              }
            }
            n498 = local read "Auto Shutter Control"() -> (w880:bool)
            n499 = And(x=w881, y=w880) -> (x .and. y?=w879:bool)
            n500 = Select(t=T5."Auto Measurement Control" ("Do Measurement"), s=w881, f=T5."No Measurement" ("Do Measurement")) -> (s? t:f=w909:T5)
          }
          frame "Grid Measurement" {
            w1063 = T25."Grid Scan" ("Measurement Type")
            w1104 = 32768 ("dimension size")
            w1114 = u16 0  # Repetition Counter
            w1115 = 0  # Grid Point Counter
            n501 = local read "Grid Points"() -> (w1116:dbl[][])
            n502 = local read "Workspace"() -> (w1073:path)
            n503 = local read "X-Position"() -> (w1127:dbl)
            n504 = local read "Y-Position"() -> (w1126:dbl)
            n505 = local read "Z-Position"() -> (w1125:dbl)
            n506 = Index Array(array=w1107) -> (element=w1108:T32)  [unwired: 1 in]
            n507 = local read "CFD Settings"() -> (w1113:T4)
            n508 = Build Array(w1127, w1126, w1125) -> (w1067:dbl[])
            n509 = Array To Cluster(array=w1067) -> (cluster=w1066:cluster{"[0]":dbl, "[1]":dbl, "[2]":dbl})
            n510 = Unbundle By Name(w1108) -> ("Dev"=w1103:i32)
            n511 = Array Size(array=w1116) -> (size(s)=w1117:i32[])
            n512 = Multiply(x="Grid Time (s)", y=1000) -> (x*y=w1065:i32)
            n513 = call "MTS_GenFileComment.vi"("Time Per Pixel [ms]"=w1065, "Measurement Type"=w1063, "error in"=w1075, "Upper Left"=w1066, "Pixels"=w1061, "Picture Size"=w1060) -> ("error out"=w1079:errorcluster, "Image Info"=w1076:T36, "Comment"=w1068:string)  [unwired: 2 in, 1 out]
            n514 = Add(x=250 ("y"), y=w1065) -> (x+y=w1099:i32)
            n515 = call "PI_MoveTo.vi"("System no."=w1129, "Target position"=w1067, "error in"=w1128, "Move"=TRUE) -> ("System no. (dup)"=w1059:i32, "error out"=w1112:errorcluster)  [unwired: 13 in, 1 out]
            n516 = Index Array(array=w1117) -> (element=w1098:i32)  [unwired: 1 in]
            n517 = call "MTS_GetNextFileName.vi"("error in (no error)"=w1079, "File Type"="ht3", "Measurement Type"="Grid", "Workspace"=w1073) -> ("error out"=w1077:errorcluster, "Next File Name"=w1071:path)  [unwired: 6 in]
            n518 = Multiply(x=w1099, y=w1098) -> (x*y=w1097:i32)
            n519 = call "HH_Set.vi"("Device List"=w1107, "CFD Settings"=w1113, "error in (no error)"=w1112) -> ("ht3 header out"=w1095:T33, "Sync Rate"=w1087:i32, "error out"=w1111:errorcluster)  [unwired: 8 in, 2 out]
            n520 = call "MTS_AddFileToWorkspace.vi"("File Name"=w1071, "File Type"=T19."pt3 File", "Measurement Type"=w1063, "File Info"=w1076, "error in (no error)"=w1077, "Tree Refnum"=w1062) -> ("File Name (dup)"=w1070:path, "error out"=w1074:errorcluster)  [unwired: 7 in, 1 out]
            n521 = Multiply(x="Repetitions", y=w1097) -> (x*y=w1094:i32)
            n522 = Bundle By Name(cluster=w1095, "AcquisitionTime (ms)"=w1094) -> (w1069:T33)
            n523 = Reciprocal(x=w1087) -> (1/x=w1089:dbl)
            n524 = Scale By Power Of 2(n=16, x=w1089) -> (x*2^n=w1086:dbl)
            n525 = call "HT3_Create.vi"("error in"=w1111, "Comment"=w1068, "ht3 Header in"=w1069, "File Path"=w1070) -> ("error out"=w1110:errorcluster, "FileHeaderPos"=w1080:T35, "refnum out"=w1093:refnum<file>)  [unwired: 5 in]
            n526 = Initialize Array(u32 0, w1104) -> (w1105:u32[])
            n527 = call "HH_Start.vi"("Device Index"=w1103, "Acq. Time"=w1094, "error in (no error)"=w1110) -> ("error out"=w1109:errorcluster)  [unwired: 11 in, 1 out]
            n528 = case shown="No Error" w1109 {
              selector: w1109 -> [w1153 w1242]
              tunnel: [w1141 w1242] -> w1092
              tunnel: w1116 -> [w1152 _]
              tunnel: w1115 -> [w1151 _]
              tunnel: w1114 -> [w1150 _]
              tunnel: w1098 -> [w1149 _]
              tunnel: "Repetitions" -> [w1148 _]
              tunnel: w1105 -> [w1147 _]
              tunnel: w1104 -> [w1146 _]
              tunnel: w1103 -> [w1145 _]
              tunnel: w1065 -> [w1144 _]
              tunnel: w1093 -> [w1143 w1239]
              tunnel: [w1139 w1241] -> w1091
              tunnel: [w1138 w1241] -> w1090
              tunnel: w1086 -> [w1137 _]
              tunnel: [w1136 0.0] -> w1085
              tunnel: [w1135 w1239] -> w1084
              tunnel: [w1134 i64 0] -> w1083
              tunnel: [w1133 u64[] [] ("Total Photon Count")] -> w1082
              tunnel: w1074 -> [w1132 w1236]
              tunnel: [w1132 w1236] -> w1081
              tunnel: w1059 -> [w1131 _]
              tunnel: TRUE ("Reset") -> [w1130 _]
              frame No Error {
                n529 = while {
                  shift-right: [w1169] -> w1142
                  shift-left: w1153 -> [w1198]
                  tunnel: w1152 -> [w1197]
                  tunnel: w1149 -> [w1193]
                  shift-right: [w1154] -> _
                  shift-left: w1151 -> [w1194]
                  shift-right: [w1186] -> _
                  shift-left: w1150 -> [w1188]
                  tunnel: w1148 -> [w1187]
                  tunnel: w1147 -> [w1184]
                  tunnel: w1146 -> [w1183]
                  tunnel: w1145 -> [w1178]
                  tunnel: w1144 -> [w1180]
                  tunnel: w1143 -> [w1179]
                  tunnel: [w1178] -> w1140
                  tunnel: [w1176] -> w1139
                  tunnel: [w1174] -> w1138
                  tunnel: w1137 -> [w1172]
                  tunnel: [w1171] -> w1136
                  tunnel: [w1167] -> w1135
                  tunnel: [w1160] -> w1134
                  tunnel: [w1159] -> w1133
                  tunnel: w1131 -> [w1158]
                  shift-right: [w1156] -> _
                  shift-left: w1130 -> [w1155]
                  stop <- w1177 stop-if-true
                  # "Trigger Puls: Special = 1 and Chan = 4"
                  # "Grid Time (ms)"
                  n530 = Index Array(array=w1197, index (row)=w1194) -> (element=w1196:dbl[])  [unwired: 1 in]
                  n531 = Increment(x=w1194) -> (x+1=w1192:i32)
                  n532 = call "PI_MoveTo.vi"("System no."=w1158, "Target position"=w1196, "error in"=w1198, "Move"=TRUE) -> ("error out"=w1185:errorcluster)  [unwired: 13 in, 2 out]
                  n533 = Equal?(x=w1193, y=w1192) -> (x = y?=w1190:bool)
                  n534 = for {
                    N: 10 -> [_]
                    tunnel: w1184 -> [w1204]
                    tunnel: w1183 -> [w1203]
                    tunnel: [w1199] -> w1181
                    tunnel: w1178 -> [w1201]
                    shift-right: [w1202] -> w1182
                    shift-left: w1185 -> [w1205]
                    n535 = Wait (ms)(milliseconds to wait=u32 10) -> (millisecond timer value=w1199:u32)
                    n536 = call "HH_FIFORead.vi"("Device Index"=w1201, "Buffer In"=w1204, "Count"=w1203, "error in (no error)"=w1205) -> ("error out"=w1202:errorcluster)  [unwired: 7 in, 4 out]
                  }
                  n537 = Boolean To (0,1)(Boolean=w1190) -> (0, 1=w1189:i16)
                  n538 = Add(x=w1189, y=w1188) -> (x+y=w1186:u16)
                  n539 = Select(t=0, s=w1190, f=w1192) -> (s? t:f=w1154:i32)
                  "Current Grid Point" <- w1154
                  n540 = Equal?(x=w1187, y=w1186) -> (x = y?=w1175:bool)
                  n541 = while {
                    tunnel: w1178 -> [w1234]
                    tunnel: w1184 -> [w1233]
                    tunnel: w1183 -> [w1232]
                    shift-right: [w1223] -> w1170
                    shift-left: w1182 -> [w1235]
                    shift-right: [FALSE ("Reset")] -> w1156
                    shift-left: w1155 -> [w1228]
                    tunnel: [w1225] -> w1176
                    tunnel: [w1216] -> w1174
                    tunnel: w1179 -> [w1220]
                    tunnel: [w1219] -> w1168
                    tunnel: [w1218] -> w1161
                    tunnel: [w1217] -> w1173
                    tunnel: [w1211] -> w1159
                    tunnel: w1181 -> [w1210]
                    tunnel: w1180 -> [w1208]
                    stop <- w1231 stop-if-true
                    n542 = call "HH_FIFORead.vi"("Device Index"=w1234, "Buffer In"=w1233, "Count"=w1232, "error in (no error)"=w1235) -> ("OK"=w1226:bool, "Buffer Out"=w1221:u32[], "Data Count"=w1222:i32, "FiFo Overrun"=w1225:bool, "error out"=w1224:errorcluster)  [unwired: 7 in]
                    n543 = Wait (ms)(milliseconds to wait=u32 10) -> (millisecond timer value=w1206:u32)
                    n544 = local write "FiFo Overrun"(w1225) -> ()
                    n545 = local read "Global Stop"() -> (w1214:bool)
                    n546 = Unbundle(w1224) -> ("status"=w1230:bool)  [unwired: 2 out]
                    n547 = Subtract(x=w1206, y=w1210) -> (x-y=w1209:u32)
                    n548 = call "HH_TraceAndHisto.vi"("Data In"=w1221, "Reset"=w1228, "Data Count"=w1222) -> ("Histograms"=w1213:i32[][], "Total Photon Count"=w1211:u64[], "Total Oveflow Count"=w1217:u64, "Num Records Total"=w1218:i64, "Traces"=w1212:i32[][])  [unwired: 8 in]
                    n549 = Greater Or Equal?(x=w1209, y=w1208) -> (x >= y?=w1207:bool)
                    n550 = local read "Stop Measurement"() -> (w1215:bool)
                    n551 = call "HT3_Write.vi"("error in"=w1224, "Data Count"=w1222, "Data in"=w1221, "refnum in"=w1220) -> ("error out"=w1223:errorcluster, "refnum out"=w1219:refnum<file>)  [unwired: 6 in]
                    n552 = local write "Histogram"(w1213) -> ()
                    n553 = local write "Trace"(w1212) -> ()
                    n554 = Compound Arithmetic op=OR(w1207, invert w1226, w1230, w1214, w1215) -> (w1231:bool)
                    n555 = Or(x=w1215, y=w1214) -> (x .or. y?=w1216:bool)
                  }
                  n556 = Logical Shift(y=25 ("x"), x=u32 68) -> (x << y=w1164:u32)
                  n557 = Build Array(w1164) -> (w1165:u32[])
                  n558 = Or(x=w1175, y=w1174) -> (x .or. y?=w1177:bool)
                  n559 = call "HT3_Write.vi"("error in"=w1170, "Data Count"=1, "Data in"=w1165, "refnum in"=w1168) -> ("error out"=w1169:errorcluster, "refnum out"=w1167:refnum<file>)  [unwired: 6 in]
                  n560 = Multiply(x=w1172, y=w1173) -> (x*y=w1171:dbl)
                  n561 = Increment(x=w1161) -> (x+1=w1160:i64)
                }
                n562 = call "HH_Stop.vi"("Device Index"=w1140, "error in (no error)"=w1142) -> ("error out"=w1141:errorcluster)  [unwired: 12 in, 1 out]
              }
              frame Error {
                w1241 = FALSE
              }
            }
            n563 = flat-sequence {
              tunnel: w1081 -> [w1266]
              tunnel: w1092 -> [w1262]
              tunnel: [w1266] -> w1119
              tunnel: [w1259] -> w1118
              tunnel: w1091 -> [w1264]
              tunnel: w1090 -> [w1252]
              tunnel: w1084 -> [w1258]
              tunnel: w1083 -> [w1257]
              tunnel: w1085 -> [w1247]
              tunnel: w1082 -> [w1246]
              tunnel: w1080 -> [w1243]
              frame #0 {
                # "Finish after Measurement"
                n564 = Or(x=w1252, y=w1264) -> (x .or. y?=w1263:bool)
                n565 = case shown="True" w1263 {
                  tunnel: w1262 -> [w1268 w1269]
                  tunnel: [w1268 w1269] -> w1260
                  tunnel: [enum16{"timeover", "manual", "overflow"}."timeover" ("Stop Reason") w1272] -> w1253
                  tunnel: w1252 -> [_ w1270]
                  frame False {
                  }
                  frame True {
                    n566 = Select(t=enum16{"timeover", "manual", "overflow"}."manual" ("Stop Reason"), s=w1270, f=enum16{"timeover", "manual", "overflow"}."overflow" ("Stop Reason")) -> (s? t:f=w1272:enum16{"timeover", "manual", "overflow"})
                  }
                }
                n567 = Multiply(x=w1247, y=1000.0) -> (x*y=w1255:dbl)
                n568 = Divide(x=w1246, y=w1247) -> (x/y=w1248:dbl[])
                n569 = To Long Integer(number=w1255) -> (32bit integer=w1254:i32)
                n570 = To Long Integer(number=w1248) -> (32bit integer=w1249:i32[])
                n571 = property on="Grid Measurement" class="Bool"("BoolText.Text"="Grid Measurement" ("Caption.Text"), "BoolText.TextColor"=u32 0 ("Boolean Text.Colors:FG Color")) -> ()  [unwired: 2 in, 2 out]
                n572 = Index Array(array=w1249, index #1=0 ("index"), index #2=1 ("index")) -> (element #1=w1245:i32, element #2=w1244:i32)
                n573 = call "HT3_Finish.vi"("Input 1 Rate"=w1244, "FileHeaderPos"=w1243, "Input 0 Rate"=w1245, "Stop Reason"=w1253, "error in"=w1260, "Num Records"=w1257, "Stop After (ms)"=w1254, "refnum in"=w1258) -> ("error out"=w1259:errorcluster)  [unwired: 3 in]
              }
            }
          }
          frame "Multi Measurement" {
            n574 = local read "X-Position"() -> (w1285:dbl)
            n575 = local read "Y-Position"() -> (w1284:dbl)
            n576 = local read "Z-Position"() -> (w1283:dbl)
            n577 = Build Array(w1285, w1284, w1283) -> (w1282:dbl[])
            n578 = call "PI_MoveTo.vi"("System no."=w1287, "Target position"=w1282, "error in"=w1286, "Move"=TRUE) -> ("System no. (dup)"=w1279:i32, "error out"=w1280:errorcluster)  [unwired: 13 in, 1 out]
          }
          frame "Save Color Image" {
            n579 = local read "Active pt3"() -> (w1296:path)
            n580 = call "MTS_GetFileFromWS.vi"(".pt3 File Name"=w1296) -> ("File Header"=w1295:T24)  [unwired: 9 in, 1 out]
            n581 = Unbundle By Name(w1295) -> ("Measurement Type"=w1294:T25, "Pixels"=w1291:i32[])
            n582 = Equal?(x=T30."Image File" ("Measurement Type"), y=w1294) -> (x = y?=w1292:bool)
            n583 = control-ref of="WS File Tree"() -> (w1297:refnum<vi>)
            n584 = case shown="True" w1292 {
              tunnel: w1302 -> [w1303 w1332]
              tunnel: w1296 -> [_ w1331]
              tunnel: w1296 -> [_ w1314]
              tunnel: [w1303 w1304] -> w1301
              tunnel: w1297 -> [_ w1311]
              tunnel: w1291 -> [_ w1310]
              frame False {
              }
              frame True {
                # "Image Intensity Array"
                # "Image Intensity Array"
                n585 = call "HT3_Open.vi"("error in"=w1332, "File Path"=w1331) -> ("error out"=w1324:errorcluster, "Header"=w1328:T37, "refnum out"=w1330:refnum<file>)  [unwired: 3 in, 4 out]
                n586 = Index Array(array=w1310, index #2=1 ("index")) -> (element #1=w1307:i32, element #2=w1308:i32)  [unwired: 1 in]
                n587 = Unbundle By Name(w1328) -> ()  [unwired: 15 out]
                n588 = Initialize Array(0 ("element"), w1307, w1308) -> (w1326:i32[][])
                n589 = while {
                  tunnel: w1330 -> [w1358]
                  shift-right: [FALSE ("Start From Top")] -> _
                  shift-left: TRUE ("Start From Top") -> [w1352]
                  shift-right: [w1351] -> w1323
                  shift-left: w1324 -> [w1346]
                  tunnel: [w1350] -> w1322
                  tunnel: w1326 -> [w1349]
                  tunnel: [w1348] -> w1325
                  tunnel: [w1347] -> _
                  stop <- w1355 stop-if-true
                  n590 = call "HT3_Read.vi"("Start From Top"=w1352, "error in"=w1346, "Data count"=10000, "refnum in"=w1358) -> ("error out"=w1351:errorcluster, "Data out"=w1354:u32[], "refnum out"=w1350:refnum<file>, "EOF?"=w1355:bool)  [unwired: 4 in]
                  n591 = Array Size(array=w1354) -> (size(s)=w1353:i32)
                  n592 = call "HH_ToImageOffline.vi"("Data In"=w1354, "Reset"=w1352, "Image Array In"=w1349, "Data Count"=w1353) -> ("Image Array Out"=w1347:i32[][], "Histograms"=w1348:i32[][])  [unwired: 2 in, 8 out]
                }
                n593 = call "MTS_SelectTCSPCBinning.vi"("Histograms in"=w1325) -> ("TCSPC Binning"=w1318:i32[][], "Colors"=w1312:u32[], "Active"=w1313:bool[])  [unwired: 1 in, 7 out]
                n594 = Initialize Array(0 ("element"), 4 ("dimension size"), w1307, w1308) -> (w1319:i32[][][])
                n595 = while {
                  tunnel: w1322 -> [w1345]
                  shift-right: [FALSE ("Start From Top")] -> _
                  shift-left: TRUE ("Start From Top") -> [w1339]
                  shift-right: [w1338] -> w1316
                  shift-left: w1323 -> [w1334]
                  tunnel: [w1337] -> w1305
                  tunnel: w1319 -> [w1336]
                  tunnel: [w1335] -> w1315
                  tunnel: w1318 -> [w1333]
                  stop <- w1342 stop-if-true
                  n596 = call "HT3_Read.vi"("Start From Top"=w1339, "error in"=w1334, "Data count"=10000, "refnum in"=w1345) -> ("error out"=w1338:errorcluster, "Data out"=w1341:u32[], "refnum out"=w1337:refnum<file>, "EOF?"=w1342:bool)  [unwired: 4 out]
                  n597 = Array Size(array=w1341) -> (size(s)=w1340:i32)
                  n598 = call "HH_ToColorImage.vi"("Data In"=w1341, "Reset"=w1339, "Image Array In"=w1336, "Data Count"=w1340, "TCSPC Binning"=w1333) -> ("Image Array Out"=w1335:i32[][][])  [unwired: 2 in, 8 out]
                }
                n599 = call "MTS_SaveColorImagePng.vi"("Tree Refnum"=w1311, ".pt3 File Name"=w1314, "error in"=w1316, "Colors"=w1312, "Active"=w1313, "Image"=w1315) -> ("error out"=w1306:errorcluster)  [unwired: 5 in]
                n600 = Close File(refnum=w1305, error in=w1306) -> (error out=w1304:errorcluster)  [unwired: 1 out]
              }
            }
          }
          frame "Find Single Mol." {
            n601 = local read "Active pt3"() -> (w1373:path)
            n602 = call "MTS_GetFileFromWS.vi"(".pt3 File Name"=w1373) -> ("File Header"=w1372:T24)  [unwired: 9 in, 1 out]
            n603 = Unbundle By Name(w1372) -> ("Measurement Type"=w1371:T25, "Pixels"=w1368:i32[], "Picture Size"=w1367:dbl[], "Upper Left"=w1366:T26, "Scan Axis"=w1365:enum32{"x-y", "x-z", "y-z"})
            n604 = call "MTS_ScannerXYZToImageXY.vi"("Axis"=w1365, "Scanner XYZ"=w1366) -> ("Image Y"=w1363:dbl, "Image X"=w1364:dbl)
            n605 = Equal?(x=T30."Image File" ("Measurement Type"), y=w1371) -> (x = y?=w1369:bool)
            n606 = case shown="True" w1369 {
              tunnel: w1378 -> [w1380 w1407]
              tunnel: w1373 -> [_ _]
              tunnel: w1373 -> [_ _]
              tunnel: [w1380 w1381] -> w1377
              tunnel: w1368 -> [_ w1414]
              tunnel: w1367 -> [_ w1413]
              tunnel: w1364 -> [_ w1401]
              tunnel: w1363 -> [_ w1402]
              tunnel: w1362 -> [w1379 w1395]
              tunnel: [w1379 w1390] -> w1361
              frame False {
              }
              frame True {
                w1412 = 1 ("index")
                # "Gauss Width"
                # "Pixel Size [um]"
                n607 = Index Array(array=w1414, index #2=w1412) -> (element #1=w1410:i32, element #2=w1405:i32)  [unwired: 1 in]
                n608 = Index Array(array=w1413, index #2=w1412) -> (element #1=w1411:dbl, element #2=w1404:dbl)  [unwired: 1 in]
                n609 = local read "Image"() -> (w1394:i32[][])
                n610 = Divide(x=w1411, y=w1410) -> (x/y=w1398:dbl)
                n611 = Divide(x=w1404, y=w1405) -> (x/y=w1403:dbl)
                n612 = Reciprocal(x=w1398) -> (1/x=w1397:dbl)
                n613 = To Double Precision Float(number=w1394) -> (double precision float=w1406:dbl[][])
                n614 = Multiply(x=w1397, y="psf width [um]") -> (x*y=w1408:dbl)
                n615 = script code="mask = GenGauss2D(gw);\n[err, bim, cim, sim, yc, xc, bc, cc, sc, len, imm] = FindPatternCP(Image, mask, [], [], [], 1.5);\nxc = xc - 1;\nyc = yc - 1;"("??"=w1407, "gw"=w1408, "Image"=w1406) -> ("??"=w1396:errorcluster, "xc"=w1385:dbl[], "yc"=w1384:dbl[])
                n616 = Multiply(x=w1398, y=w1385) -> (x*y=w1400:dbl[])
                n617 = Multiply(x=w1384, y=w1403) -> (x*y=w1399:dbl[])
                n618 = Add(x=w1401, y=w1400) -> (x+y=w1387:dbl[])
                n619 = Add(x=w1399, y=w1402) -> (x+y=w1386:dbl[])
                n620 = call "MTS_IntensityArrayToImage.vi"(0:"Image"=w1395, 1:"Image"=w1394, "error in (no error)"=w1396, "Log Scale"=TRUE) -> ("Image Out"=w1391:T3, "error out"=w1392:errorcluster)  [unwired: 10 in]
                n621 = for {
                  shift-right: [w1421] -> w1390
                  shift-left: w1391 -> [w1422]
                  tunnel: w1385 -> [w1420] mode=indexing
                  tunnel: w1384 -> [w1419] mode=indexing
                  shift-right: [w1423] -> w1382
                  shift-left: w1392 -> [w1424]
                  tunnel: u32 16738560 -> [w1418]
                  tunnel: 3.0 ("x") -> [w1417]
                  n622 = call "MTS_DrawCrossIMAQIamge.vi"("Image"=w1422, "Size"=w1417, "Color"=w1418, "X"=w1420, "Y"=w1419, "error in (no error)"=w1424) -> ("Image Out"=w1421:T3, "error out"=w1423:errorcluster)  [unwired: 8 in]
                }
                "AM image" <- w1390
                n623 = Build Array(w1387, w1386, w1385, w1384) -> (→"Pattern":dbl[][])
                n624 = flat-sequence {
                  tunnel: w1382 -> [w1415]
                  tunnel: [w1415] -> w1381
                  frame #0 {
                    n625 = local write "ShowTab"(T2."Auto Measurement" ("ShowTab")) -> ()
                  }
                }
              }
            }
          }
          frame "Auto Measurement Control" {
            # "Init"
            n626 = local read "Pattern"() -> (w1436:dbl[][])
            n627 = local read "NxtAutMesPoint"() -> (w1429:i32)
            n628 = Index Array(array=w1436, index (row)=0) -> (element=w1443:dbl[])  [unwired: 1 in]
            n629 = Less Than 0?(x=w1429) -> (x < 0?=w1441:bool)
            n630 = case shown="True" w1441 {
              tunnel: w1443 -> [_ w1478]
              tunnel: w1442 -> [w1469 w1473]
              tunnel: [w1469 w1472] -> w1439
              tunnel: [w1468 w1470] -> w1428
              frame False {
                n631 = local read "Auto Measure Points"() -> (w1468:i32)
              }
              frame True {
                n632 = Array Size(array=w1478) -> (size(s)=w1470:i32)
                "Auto Measure Points" <- w1470
                n633 = Number To Decimal String(number=w1470) -> (decimal integer string=w1475:string)  [unwired: 1 in]
                n634 = Concatenate Strings("Point 1 / " ("Caption.Text"), w1475) -> (w1474:string)
                n635 = property on="Auto Meas Progress" class="Slide (strict)"(error in=w1473, "Scale.Minimum"=0.0 ("Scale.Range:Minimum"), "Scale.Maximum"=w1470, "Value"=1 ("Auto Meas Progress"), "Caption.Text"=w1474) -> (error out=w1472:errorcluster)  [unwired: 1 in, 1 out]
              }
            }
            n636 = Increment(x=w1429) -> (x+1=w1427:i32)
            "NxtAutMesPoint" <- w1427
            n637 = Greater Or Equal?(x=w1427, y=w1428) -> (x >= y?=w1440:bool)
            n638 = Increment(x=w1427) -> (x+1=w1426:i32)
            n639 = Index Array(array=w1436, index (row) #1=2 ("index (row)"), index (col) #1=w1427, index (row) #2=3 ("index (row)"), index (col) #2=w1427) -> (element #1=w1433:dbl, element #2=w1432:dbl)
            n640 = case shown="False" w1440 {
              tunnel: w1439 -> [w1459 w1467]
              tunnel: [w1464 w1467] -> w1438
              tunnel: [T5."Auto Point" ("Do Measurement") T16."No Measurement" ("Do Measurement")] -> w1437
              tunnel: w1426 -> [w1460 _]
              tunnel: w1433 -> [w1457 _]
              tunnel: w1432 -> [w1456 _]
              tunnel: w1431 -> [w1453 w1465]
              tunnel: [w1452 w1465] -> w1430
              tunnel: w1428 -> [w1449 _]
              frame False {
                # "Prpare For Next Point"
                n641 = call "MTS_DrawCrossIMAQIamge.vi"("Image"=w1453, "Size"=3.0 ("x"), "Color"=u32 6618880, "X"=w1457, "Y"=w1456, "error in (no error)"=w1459) -> ("Image Out"=w1452:T3, "error out"=w1458:errorcluster)  [unwired: 8 in]
                n642 = Number To Decimal String(number=w1449) -> (decimal integer string=w1450:string)  [unwired: 1 in]
                n643 = Number To Decimal String(number=w1460) -> (decimal integer string=w1462:string)  [unwired: 1 in]
                n644 = Concatenate Strings("Point " ("Caption.Text"), w1462, " / " ("Caption.Text"), w1450) -> (w1461:string)
                n645 = property on="Auto Meas Progress" class="Slide (strict)"(error in=w1458, "Value"=w1460, "Caption.Text"=w1461) -> (error out=w1464:errorcluster)  [unwired: 1 in, 1 out]
                n646 = local write "AM image"(w1452) -> ()
              }
              frame True {
                # "No More Points"
              }
            }
          }
        }
      }
      frame Error {
      }
    }
    n647 = flat-sequence {
      tunnel: w589 -> [w1499]
      tunnel: [w1499] -> w588
      tunnel: w582 -> [w1494]
      tunnel: w580 -> [w1495]
      frame #0 {
        n648 = control-ref of="ShowTab"() -> (w1498:refnum<vi>)
        n649 = case shown="True" w1495 {
          frame False {
          }
          frame True {
            w1500 = TRUE ("Detector2")
            n650 = call "PCAN_CompMessage.vi"("Excitation"=FALSE, "Detector4"=w1500, "Detector3"=w1500, "Detector2"=w1500, "Detector1"=w1500) -> ("CAN_Message"=w1502:T28)  [unwired: 6 in]
            n651 = call "CAN PCI Write.vi"("CAN_Message"=w1502) -> ()  [unwired: 2 in, 1 out]
          }
        }
        n652 = Equal?(x=w1494, y=T5."No Measurement" ("Do Measurement")) -> (x = y?=w1496:bool)
        n653 = Not(x=w1496) -> (.not. x?=w1497:bool)
        n654 = case shown="True" w1496 {
          tunnel: w1498 -> [_ w1503]
          frame False {
          }
          frame True {
            n655 = call "MTS_ShowHideTabs.vi"("Action"=enum16{"Show All", "Hide Tab", "Show Tab"}."Show All", "ShowTab"=w1503) -> ()  [unwired: 8 in, 2 out]
          }
        }
        n656 = local write "Do Measurement"(w1494) -> ()
        n657 = local write "MeasRunig"(w1497) -> ()
      }
    }
    n658 = Unbundle(w586) -> ("status"=w585:bool)  [unwired: 2 out]
    n659 = local read "Global Stop"() -> (w592:bool)
    n660 = Compound Arithmetic op=OR(w585, w590, w592) -> (w591:bool)
  }
  n661 = while {
    tunnel: w8 -> [w1508]
    shift-right: [w1507] -> _
    shift-left: w10 -> [w1509]
    stop <- w1506 stop-if-true
    n662 = Wait (ms)(milliseconds to wait=u32 50) -> ()  [unwired: 1 out]
    n663 = case shown="True" "SCANNER EMERGENCY" {
      tunnel: w1508 -> [_ w1514]
      tunnel: w1509 -> [w1512 w1515]
      tunnel: [w1512 w1516] -> w1507
      frame False {
        n664 = Wait Until Next ms Multiple(millisecond multiple=u32 100) -> ()  [unwired: 1 out]
      }
      frame True {
        n665 = call "PI_Stop_Wave_Gen.vi"("System no."=w1514, "error in"=w1515) -> ("error out"=w1513:errorcluster)  [unwired: 12 in, 1 out]
        n666 = flat-sequence {
          tunnel: [w1517] -> w1516
          tunnel: w1513 -> [w1517]
          frame #0 {
            n667 = One Button Dialog(message="Emergency scanner stop appeared!!!\nCheck scanner settings before continue!!!") -> ()  [unwired: 2 out]
          }
        }
      }
    }
    n668 = local read "Global Stop"() -> (w1506:bool)
  }
  n669 = call "DT3120_CloseDevice.vi"("error in (no error)"=w26, "lpDevId"=w24) -> ("error out"=w19:errorcluster)  [unwired: 9 out]
  n670 = call "IMAQ Dispose"("Image"=w18, "error in (no error)"=w19) -> ("error out"=w17:errorcluster)  [unwired: 4 in]
  n671 = flat-sequence {
    tunnel: w17 -> [w1521]
    tunnel: [w1519] -> w16
    frame #0 {
      n672 = call "CAN PCI Close.vi"() -> ("Error Number"=w1520:u32)  [unwired: 1 in]
      n673 = call <vilib>:"Error Cluster From Error Code.vi"("error in (no error)"=w1521, "error message (\"\")"="PCAN Close Error" ("error message (\"\")"), "error code (0)"=w1520) -> ("error out"=w1519:errorcluster)  [unwired: 6 in]
    }
  }
  n674 = Merge Errors(w16, w23) -> (w22:errorcluster)
  n675 = flat-sequence {
    tunnel: w29 -> [w1523]
    tunnel: [w1523] -> w28
    frame #0 {
      n676 = local write "Global Stop"(TRUE ("Global Stop")) -> ()
    }
  }
  n677 = call "IMAQ Dispose"("Image"=w13, "error in (no error)"=w15) -> ("error out"=w14:errorcluster)  [unwired: 4 in]
  n678 = call <userlib>:"Close connection if open.vi"("System no."=w35, "error in"=w28) -> ("error out"=w34:errorcluster)  [unwired: 16 in, 1 out]
  n679 = Merge Errors(w22, w14, w34) -> (w33:errorcluster)
  n680 = call <vilib>:"Simple Error Handler.vi"("error in (no error)"=w33) -> ()  [unwired: 4 in, 5 out]
